vi "Set Test Window Topmost hacker.vi"(4 "error in (no error)":errorcluster, 7 "VI Refnum":refnum<vi>) -> (0 "error out":errorcluster, 1 "hWnd reference":T1, 2 "Window name":string, 3 "dup VI Refnum":refnum<vi>)   [LabVIEW 2011]
uses:
  SI.LIB/WIN32/WinUSER/Windows/hWnd.ctl
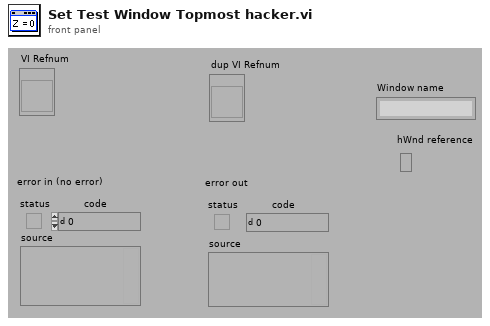
[diagram p1: front panel]
types:
  T1 = typedef "hWnd.ctl" = refnum<k1>
  T2 = enum32{"SW_SHOWDEFAULT", "SW_FORCEMINIMIZE", "SW_HIDE", "SW_MAXIMIZE", "SW_RESTORE", "SW_SHOW", "SW_SHOWMAXIMIZED", "SW_SHOWMINIMIZED", "SW_SHOWMINNOACTIVE", "SW_SHOWNA", "SW_SHOWNOACTIVATE", "SW_SHOWNORMAL"}
  T3 = cluster{"SWP_NOSIZE (x1)":bool, "SWP_NOMOVE (x2)":bool, "SWP_NOZORDER (x4)":bool, "SWP_NOREDRAW (x8)":bool, "SWP_NOACTIVATE (x10)":bool, "SWP_DRAWFRAME (x20)":bool, "SWP_SHOWWINDOW (x40)":bool, "SWP_HIDEWINDOW (x80)":bool, "SWP_NOCOPYBITS (x100)":bool, "SWP_NOOWNERZORDER (x200)":bool, "SWP_NOSENDCHANGING (x400)":bool, "SWP_DEFERERASE (x2000)":bool, "SWP_ASYNCWINDOWPOS (x4000)":bool}
  T4 = enum16{"HWND_TOP", "HWND_BOTTOM", "HWND_TOPMOST", "HWND_NOTOPMOST"}
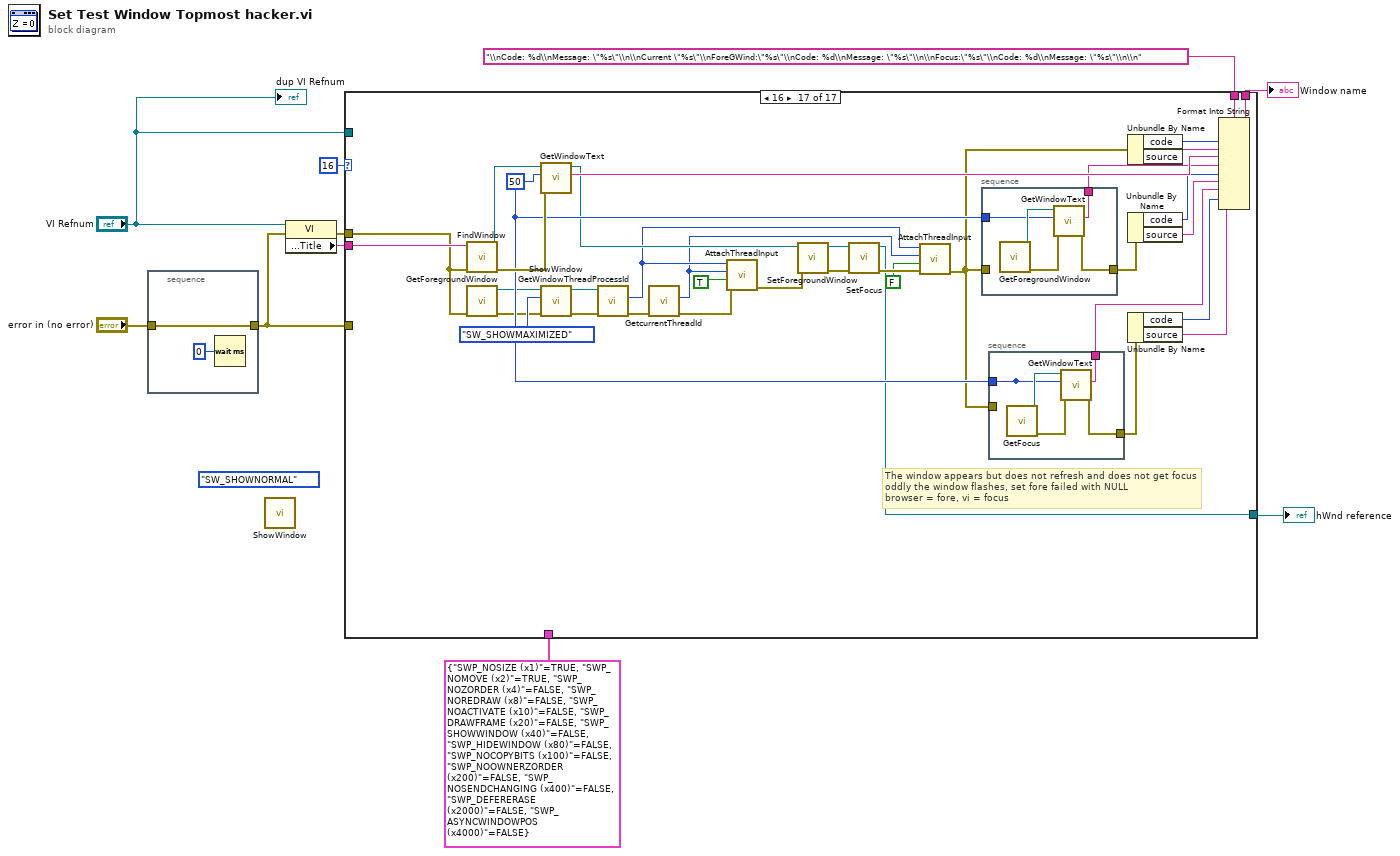
[diagram p0: block diagram]
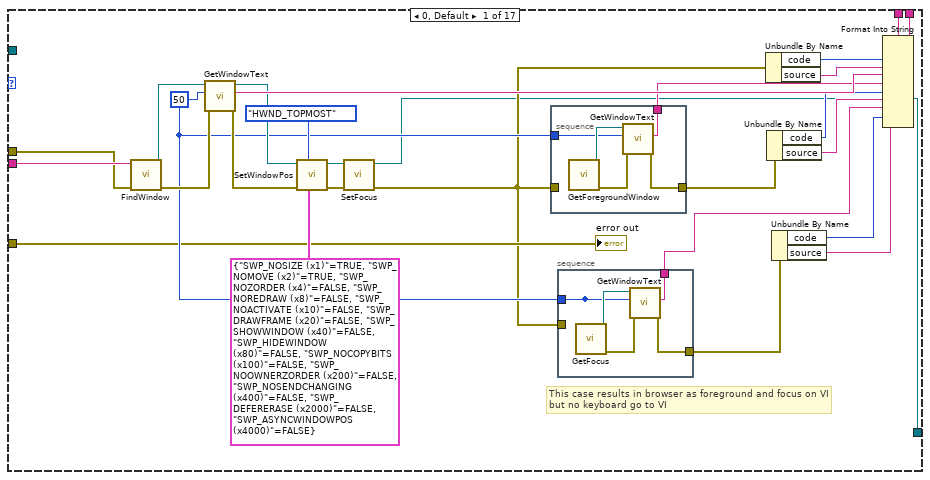
[diagram p2: hidden frame]
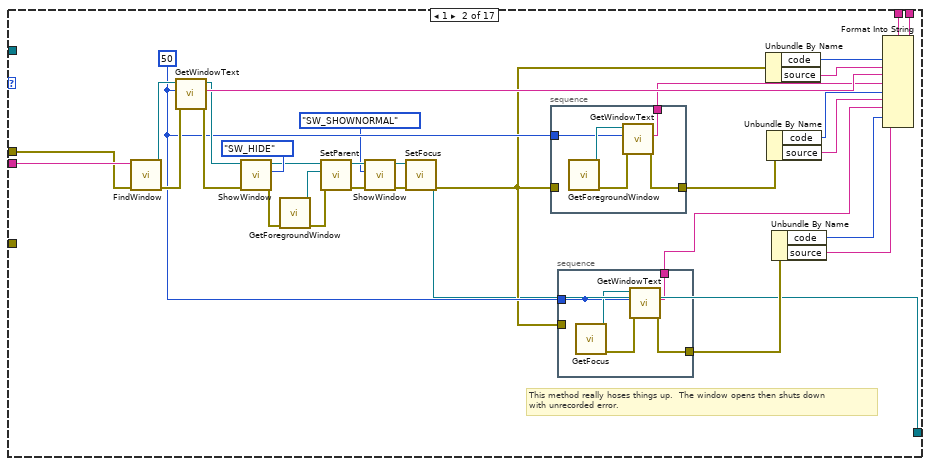
[diagram p3: hidden frame]
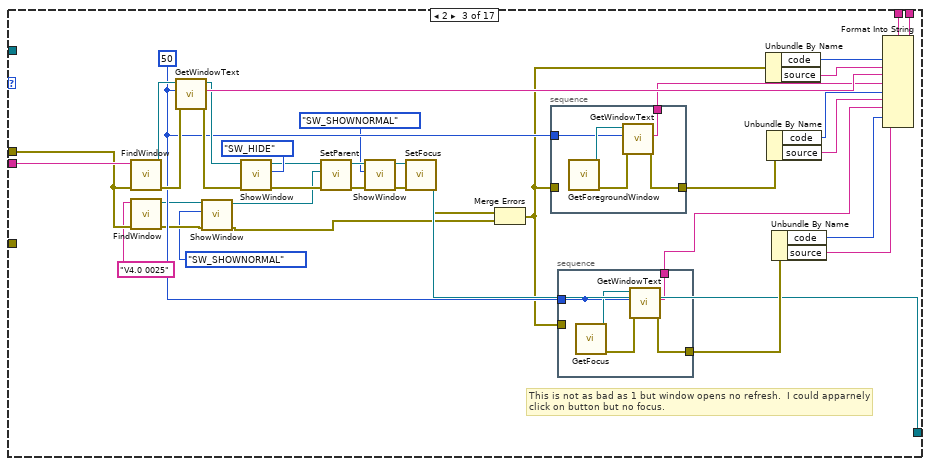
[diagram p4: hidden frame]
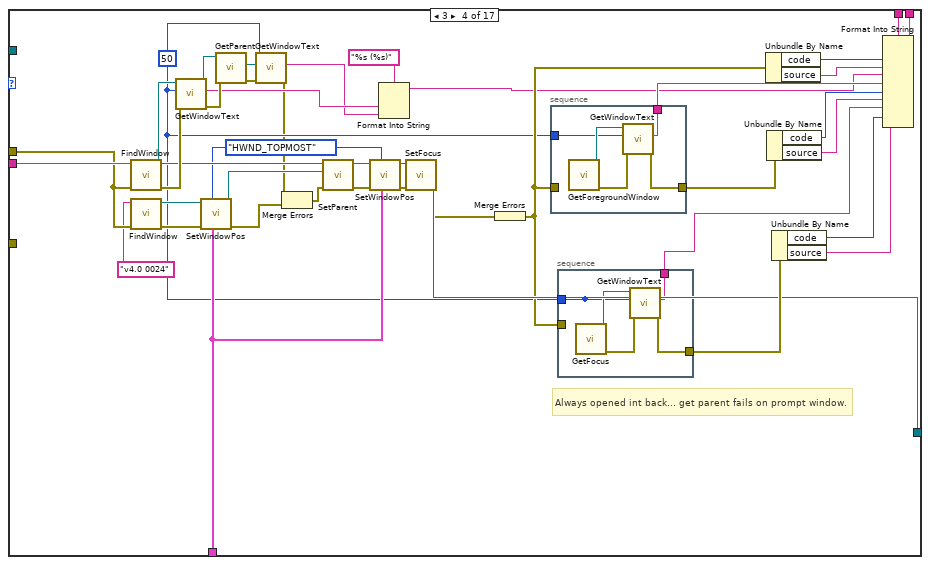
[diagram p5: hidden frame]
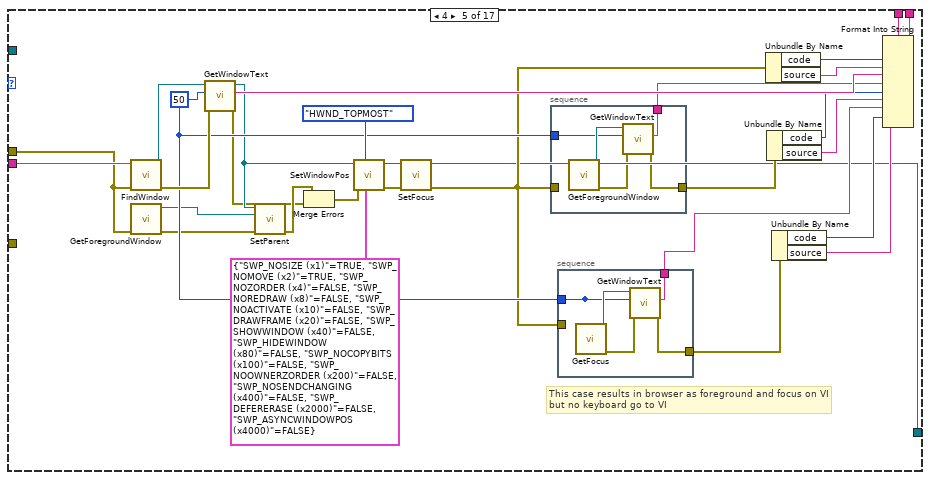
[diagram p6: hidden frame]
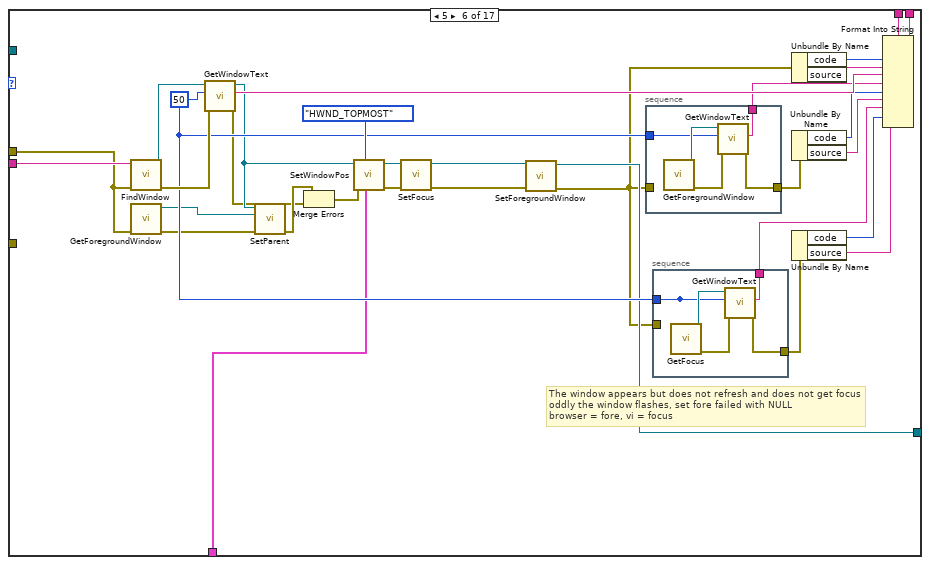
[diagram p7: hidden frame]
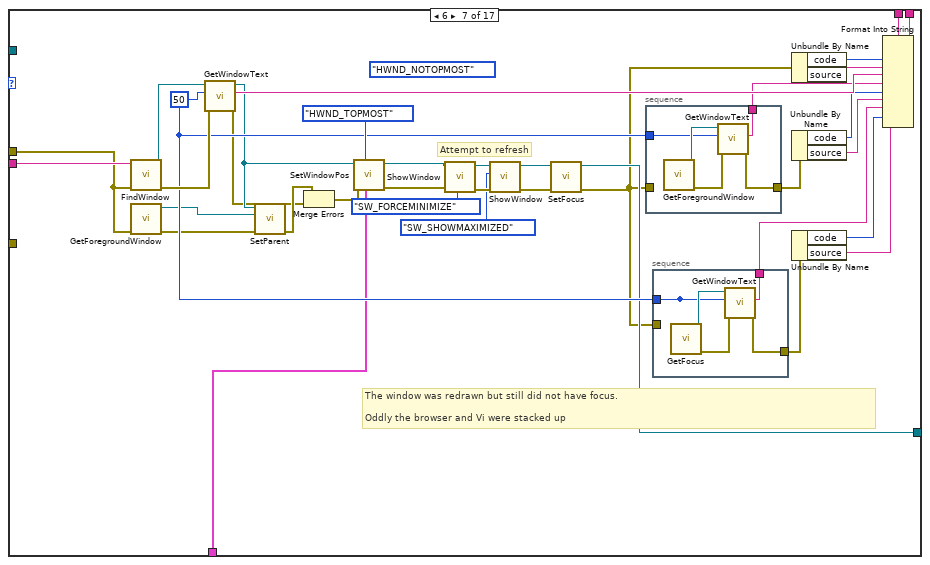
[diagram p8: hidden frame]
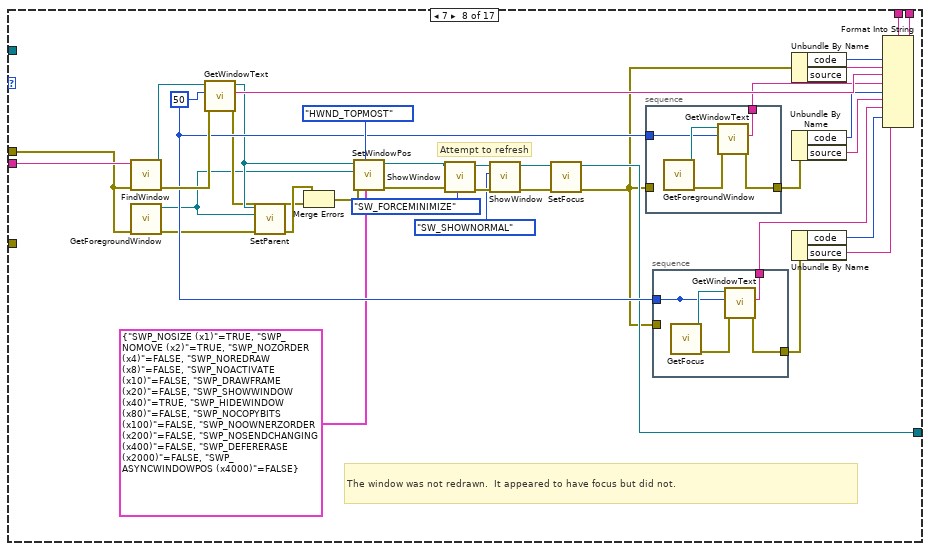
[diagram p9: hidden frame]
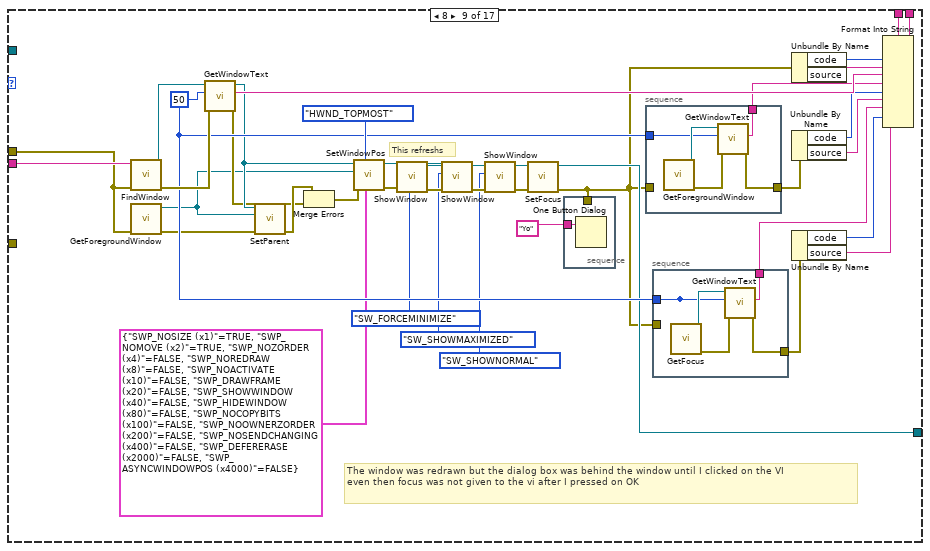
[diagram p10: hidden frame]
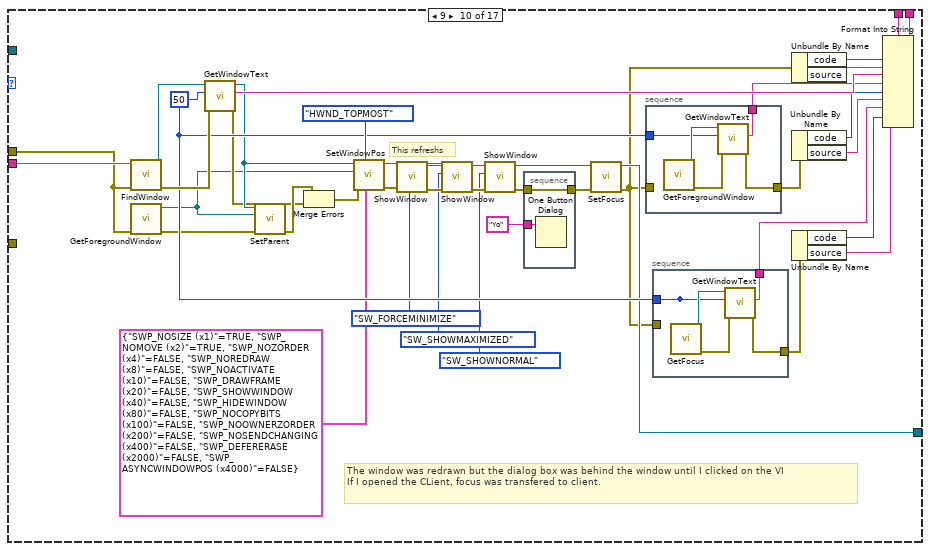
[diagram p11: hidden frame]
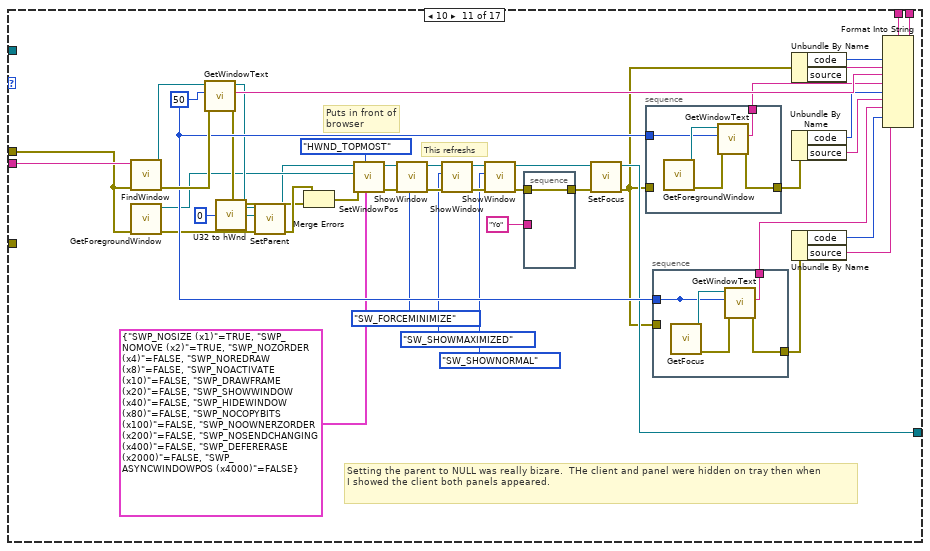
[diagram p12: hidden frame]
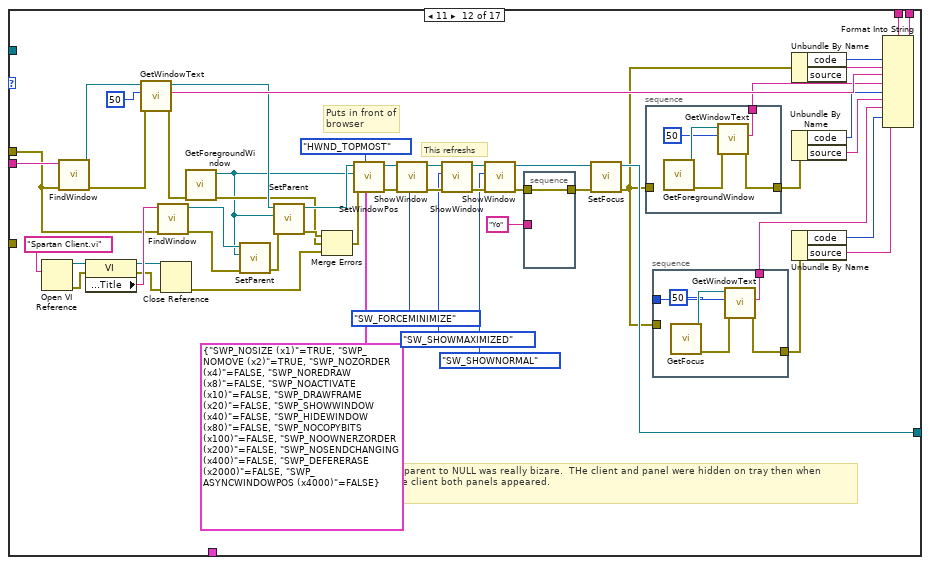
[diagram p13: hidden frame]
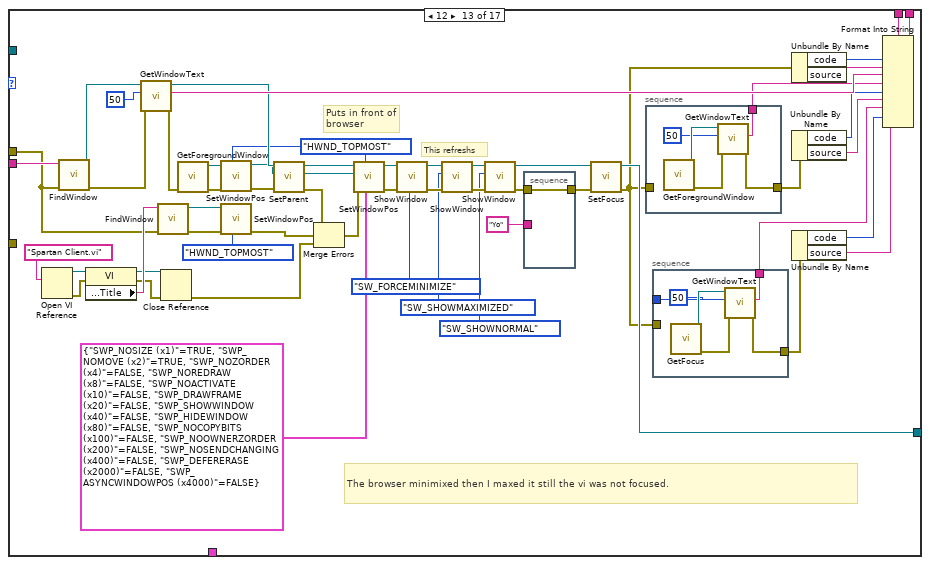
[diagram p14: hidden frame]
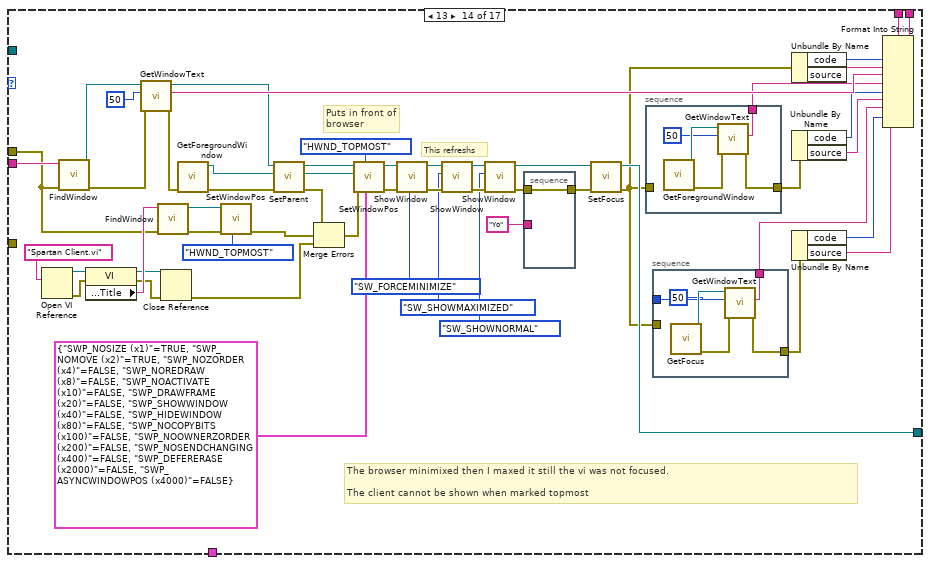
[diagram p15: hidden frame]
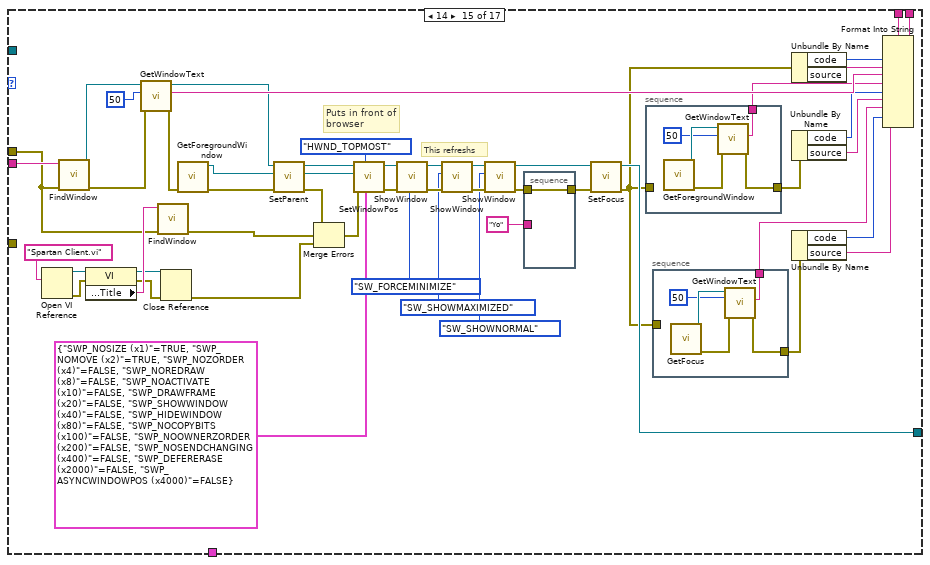
[diagram p16: hidden frame]
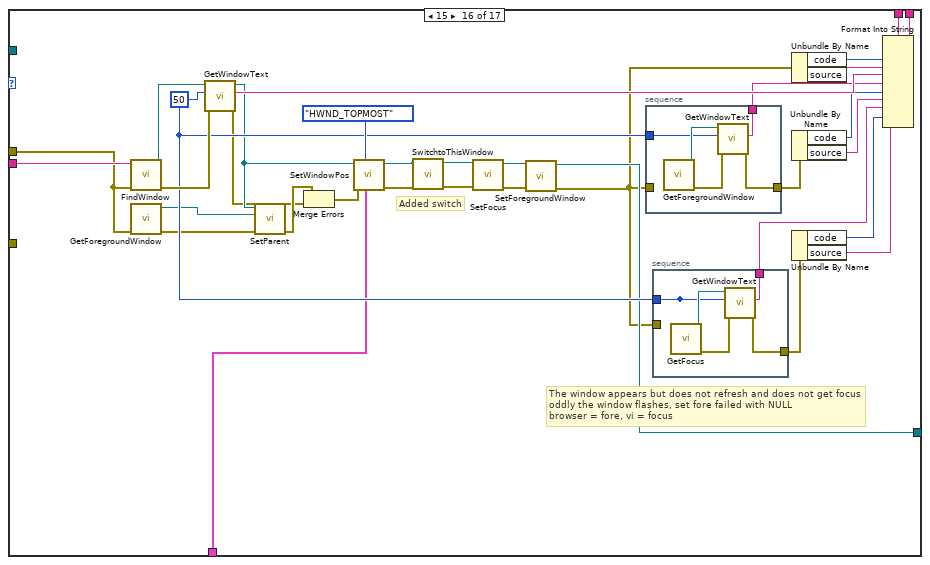
[diagram p17: hidden frame]
diagram:
  (unwired) T2."SW_SHOWNORMAL" ("nCmdShow\n(SW_SHOWNORMAL)")
  n1 = stacked-sequence {
    tunnel: "error in (no error)" -> [w12]
    tunnel: [w12] -> w5
    frame #0 {
      n2 = Wait (ms)(milliseconds to wait=u32 0) -> ()  [unwired: 1 out]
    }
  }
  n3 = call "ShowWindow.vi"() -> ()  [unwired: 4 in, 8 out]
  n4 = property class="VI"(reference="VI Refnum", error in=w5) -> (error out=w7:errorcluster, "Front Panel Window:Title"=w10:string)  [unwired: 1 out]
  n5 = case shown="16" 16 ("nMaxCount") {
    tunnel: w10 -> [w38 w81 w128 w179 w218 w261 w307 w353 w403 w455 w511 w574 w640 w704 w765 w810 w856]
    tunnel: "\\nCode: %d\\nMessage: \"%s\"\\n\\nCurrent \"%s\"\\nForeGWind:\"%s\"\\nCode: %d\\nMessage: \"%s\"\\n\\nFocus:\"%s\"\\nCode: %d\\nMessage: \"%s\"\\n\\n" ("format string") -> [w37 w80 w127 w178 w217 w260 w306 w352 w402 w454 w510 w573 w639 w703 w764 w809 w855]
    tunnel: [w36 w79 w126 w177 w216 w259 w305 w351 w401 w453 w509 w572 w638 w702 w763 w808 w854] -> w8
    tunnel: w7 -> [w34 w78 w101 w164 w196 w241 w289 w335 w385 w437 w493 w533 w601 w665 w726 w792 w839]
    tunnel: w5 -> [w15 _ _ _ _ _ _ _ _ _ _ _ _ _ _ _ _]
    tunnel: [w13 w60 w109 w165 w197 w231 w274 w322 w373 w425 w481 w547 w615 w679 w740 w782 w821] -> w4
    tunnel: T3 {"SWP_NOSIZE (x1)"=TRUE, "SWP_NOMOVE (x2)"=TRUE, "SWP_NOZORDER (x4)"=FALSE, "SWP_NOREDRAW (x8)"=FALSE, "SWP_NOACTIVATE (x10)"=FALSE, "SWP_DRAWFRAME (x20)"=FALSE, "SWP_SHOWWINDOW (x40)"=FALSE, "SWP_HIDEWINDOW (x80)"=FALSE, "SWP_NOCOPYBITS (x100)"=FALSE, "SWP_NOOWNERZORDER (x200)"=FALSE, "SWP_NOSENDCHANGING (x400)"=FALSE, "SWP_DEFERERASE (x2000)"=FALSE, "SWP_ASYNCWINDOWPOS (x4000)"=FALSE} ("Flags") -> [_ _ _ w151 _ w234 w282 _ _ _ _ _ _ _ _ w785 _]
    tunnel: "VI Refnum" -> [_ _ _ _ _ _ _ _ _ _ _ _ _ _ _ _ _]
    frame 0, Default {
      w21 = 50 ("nMaxCount")
      # "This case results in browser as foreground and focus on VI\nbut no keyboard go to VI"
      n6 = call "FindWindow.vi"("error in (no error)"=w34, "window name (\"\")"=w38) -> ("error out"=w30:errorcluster, "hWnd"=w25:T1)  [unwired: 6 out]
      n7 = call "GetWindowText.vi"("error in (no error)"=w30, "nMaxCount"=w21, "hWnd (NULL)"=w25) -> ("error out"=w29:errorcluster, "window text"=w31:string, "dup hWnd"=w27:T1)  [unwired: 6 out]
      n8 = call "SetWindowPos.vi"("Flags"=T3 {"SWP_NOSIZE (x1)"=TRUE, "SWP_NOMOVE (x2)"=TRUE, "SWP_NOZORDER (x4)"=FALSE, "SWP_NOREDRAW (x8)"=FALSE, "SWP_NOACTIVATE (x10)"=FALSE, "SWP_DRAWFRAME (x20)"=FALSE, "SWP_SHOWWINDOW (x40)"=FALSE, "SWP_HIDEWINDOW (x80)"=FALSE, "SWP_NOCOPYBITS (x100)"=FALSE, "SWP_NOOWNERZORDER (x200)"=FALSE, "SWP_NOSENDCHANGING (x400)"=FALSE, "SWP_DEFERERASE (x2000)"=FALSE, "SWP_ASYNCWINDOWPOS (x4000)"=FALSE}, "hWndInsertAfterALT\n(HWND_TOP)"=T4."HWND_TOPMOST" ("hWndInsertAfterALT\n(HWND_TOP)"), "error in (no error)"=w29, "hWnd (NULL)"=w27) -> ("error out"=w28:errorcluster, "dup hWnd"=w26:T1)  [unwired: 2 in, 4 out]
      n9 = call "SetFocus.vi"("error in (no error)"=w28, "hWnd (NULL)"=w26) -> ("error out"=w14:errorcluster, "dup hWnd"=w13:T1)  [unwired: 8 out]
      n10 = stacked-sequence {
        tunnel: w21 -> [w48]
        tunnel: [w46] -> w22
        tunnel: [w45] -> w16
        tunnel: w14 -> [_]
        frame #0 {
          n11 = call "GetForegroundWindow.vi"() -> ("error out"=w47:errorcluster, "dup hWnd"=w49:T1)  [unwired: 1 in, 9 out]
          n12 = call "GetWindowText.vi"("error in (no error)"=w47, "nMaxCount"=w48, "hWnd (NULL)"=w49) -> ("error out"=w45:errorcluster, "window text"=w46:string)  [unwired: 7 out]
        }
      }
      n13 = stacked-sequence {
        tunnel: [w40] -> _
        tunnel: [w42] -> w17
        tunnel: [w41] -> w20
        tunnel: w21 -> [w40]
        tunnel: w14 -> [_]
        frame #0 {
          n14 = call "GetFocus.vi"() -> ("error out"=w43:errorcluster, "dup hWnd"=w44:T1)  [unwired: 1 in, 9 out]
          n15 = call "GetWindowText.vi"("error in (no error)"=w43, "nMaxCount"=w40, "hWnd (NULL)"=w44) -> ("error out"=w41:errorcluster, "window text"=w42:string)  [unwired: 7 out]
        }
      }
      n16 = Unbundle By Name(w14) -> ("code"=w33:i32, "source"=w32:string)
      n17 = Unbundle By Name(w16) -> ("code"=w24:i32, "source"=w23:string)
      n18 = Unbundle By Name(w20) -> ("code"=w18:i32, "source"=w19:string)
      n19 = Format Into String(format string=w37, w33, w32, w31, w22, w24, w23, w17, w18, w19) -> (resulting string=w36:string)  [unwired: 2 in, 1 out]
      "error out" <- w15
    }
    frame 1 {
      w67 = 50 ("nMaxCount")
      # "This method really hoses things up.  The window opens then shuts down\nwith unrecorded error."
      n20 = call "FindWindow.vi"("error in (no error)"=w78, "window name (\"\")"=w81) -> ("error out"=w74:errorcluster, "hWnd"=w71:T1)  [unwired: 6 out]
      n21 = call "GetWindowText.vi"("error in (no error)"=w74, "nMaxCount"=w67, "hWnd (NULL)"=w71) -> ("error out"=w73:errorcluster, "window text"=w75:string, "dup hWnd"=w72:T1)  [unwired: 6 out]
      n22 = call "ShowWindow.vi"("error in (no error)"=w73, "nCmdShow\n(SW_SHOWNORMAL)"=T2."SW_HIDE" ("nCmdShow\n(SW_SHOWNORMAL)"), "hWnd (NULL)"=w72) -> ("error out"=w58:errorcluster, "dup hWnd"=w57:T1)  [unwired: 1 in, 6 out]
      n23 = call "GetForegroundWindow.vi"("error in (no error)"=w58) -> ("error out"=w55:errorcluster, "dup hWnd"=w56:T1)  [unwired: 9 out]
      n24 = call "SetParent.vi"("error in (no error)"=w55, "hWndParent (NULL)"=w56, "hWndChild (NULL)"=w57) -> ("error out"=w54:errorcluster, "dup hWndChild"=w53:T1)  [unwired: 7 out]
      n25 = call "ShowWindow.vi"("error in (no error)"=w54, "nCmdShow\n(SW_SHOWNORMAL)"=T2."SW_SHOWNORMAL" ("nCmdShow\n(SW_SHOWNORMAL)"), "hWnd (NULL)"=w53) -> ("error out"=w51:errorcluster, "dup hWnd"=w52:T1)  [unwired: 1 in, 6 out]
      n26 = call "SetFocus.vi"("error in (no error)"=w51, "hWnd (NULL)"=w52) -> ("error out"=w61:errorcluster, "dup hWnd"=w60:T1)  [unwired: 8 out]
      n27 = stacked-sequence {
        tunnel: w67 -> [w90]
        tunnel: [w88] -> w68
        tunnel: [w87] -> w62
        tunnel: w61 -> [_]
        frame #0 {
          n28 = call "GetForegroundWindow.vi"() -> ("error out"=w89:errorcluster, "dup hWnd"=w91:T1)  [unwired: 1 in, 9 out]
          n29 = call "GetWindowText.vi"("error in (no error)"=w89, "nMaxCount"=w90, "hWnd (NULL)"=w91) -> ("error out"=w87:errorcluster, "window text"=w88:string)  [unwired: 7 out]
        }
      }
      n30 = stacked-sequence {
        tunnel: [w82] -> _
        tunnel: [w84] -> w63
        tunnel: [w83] -> w66
        tunnel: w67 -> [w82]
        tunnel: w61 -> [_]
        frame #0 {
          n31 = call "GetFocus.vi"() -> ("error out"=w85:errorcluster, "dup hWnd"=w86:T1)  [unwired: 1 in, 9 out]
          n32 = call "GetWindowText.vi"("error in (no error)"=w85, "nMaxCount"=w82, "hWnd (NULL)"=w86) -> ("error out"=w83:errorcluster, "window text"=w84:string)  [unwired: 7 out]
        }
      }
      n33 = Unbundle By Name(w61) -> ("code"=w77:i32, "source"=w76:string)
      n34 = Unbundle By Name(w62) -> ("code"=w70:i32, "source"=w69:string)
      n35 = Unbundle By Name(w66) -> ("code"=w64:i32, "source"=w65:string)
      n36 = Format Into String(format string=w80, w77, w76, w75, w68, w70, w69, w63, w64, w65) -> (resulting string=w79:string)  [unwired: 2 in, 1 out]
    }
    frame 2 {
      w115 = 50 ("nMaxCount")
      # "This is not as bad as 1 but window opens no refresh.  I could apparnely\nclick on button but no focus."
      n37 = call "FindWindow.vi"("error in (no error)"=w101, "window name (\"\")"=w128) -> ("error out"=w122:errorcluster, "hWnd"=w119:T1)  [unwired: 6 out]
      n38 = call "FindWindow.vi"("error in (no error)"=w101, "window name (\"\")"="V4.0 0025") -> ("error out"=w97:errorcluster, "hWnd"=w98:T1)  [unwired: 6 out]
      n39 = call "GetWindowText.vi"("error in (no error)"=w122, "nMaxCount"=w115, "hWnd (NULL)"=w119) -> ("error out"=w121:errorcluster, "window text"=w123:string, "dup hWnd"=w120:T1)  [unwired: 6 out]
      n40 = call "ShowWindow.vi"("error in (no error)"=w97, "nCmdShow\n(SW_SHOWNORMAL)"=T2."SW_SHOWNORMAL" ("nCmdShow\n(SW_SHOWNORMAL)"), "hWnd (NULL)"=w98) -> ("error out"=w93:errorcluster, "dup hWnd"=w95:T1)  [unwired: 1 in, 6 out]
      n41 = call "ShowWindow.vi"("error in (no error)"=w121, "nCmdShow\n(SW_SHOWNORMAL)"=T2."SW_HIDE" ("nCmdShow\n(SW_SHOWNORMAL)"), "hWnd (NULL)"=w120) -> ("error out"=w99:errorcluster, "dup hWnd"=w107:T1)  [unwired: 1 in, 6 out]
      n42 = call "SetParent.vi"("error in (no error)"=w99, "hWndParent (NULL)"=w95, "hWndChild (NULL)"=w107) -> ("error out"=w106:errorcluster, "dup hWndChild"=w105:T1)  [unwired: 7 out]
      n43 = call "ShowWindow.vi"("error in (no error)"=w106, "nCmdShow\n(SW_SHOWNORMAL)"=T2."SW_SHOWNORMAL" ("nCmdShow\n(SW_SHOWNORMAL)"), "hWnd (NULL)"=w105) -> ("error out"=w103:errorcluster, "dup hWnd"=w104:T1)  [unwired: 1 in, 6 out]
      n44 = call "SetFocus.vi"("error in (no error)"=w103, "hWnd (NULL)"=w104) -> ("error out"=w94:errorcluster, "dup hWnd"=w109:T1)  [unwired: 8 out]
      n45 = Merge Errors(w94, w93) -> (w92:errorcluster)
      n46 = stacked-sequence {
        tunnel: w115 -> [w137]
        tunnel: [w135] -> w116
        tunnel: [w134] -> w110
        tunnel: w92 -> [_]
        frame #0 {
          n47 = call "GetForegroundWindow.vi"() -> ("error out"=w136:errorcluster, "dup hWnd"=w138:T1)  [unwired: 1 in, 9 out]
          n48 = call "GetWindowText.vi"("error in (no error)"=w136, "nMaxCount"=w137, "hWnd (NULL)"=w138) -> ("error out"=w134:errorcluster, "window text"=w135:string)  [unwired: 7 out]
        }
      }
      n49 = stacked-sequence {
        tunnel: [w129] -> _
        tunnel: [w131] -> w111
        tunnel: [w130] -> w114
        tunnel: w115 -> [w129]
        tunnel: w92 -> [_]
        frame #0 {
          n50 = call "GetFocus.vi"() -> ("error out"=w132:errorcluster, "dup hWnd"=w133:T1)  [unwired: 1 in, 9 out]
          n51 = call "GetWindowText.vi"("error in (no error)"=w132, "nMaxCount"=w129, "hWnd (NULL)"=w133) -> ("error out"=w130:errorcluster, "window text"=w131:string)  [unwired: 7 out]
        }
      }
      n52 = Unbundle By Name(w92) -> ("code"=w125:i32, "source"=w124:string)
      n53 = Unbundle By Name(w110) -> ("code"=w118:i32, "source"=w117:string)
      n54 = Unbundle By Name(w114) -> ("code"=w112:i32, "source"=w113:string)
      n55 = Format Into String(format string=w127, w125, w124, w123, w116, w118, w117, w111, w112, w113) -> (resulting string=w126:string)  [unwired: 2 in, 1 out]
    }
    frame 3 {
      w152 = T4."HWND_TOPMOST" ("hWndInsertAfterALT\n(HWND_TOP)")
      w147 = 50 ("nMaxCount")
      # "Always opened int back... get parent fails on prompt window."
      n56 = call "FindWindow.vi"("error in (no error)"=w164, "window name (\"\")"=w179) -> ("error out"=w174:errorcluster, "hWnd"=w159:T1)  [unwired: 6 out]
      n57 = call "FindWindow.vi"("error in (no error)"=w164, "window name (\"\")"="v4.0 0024") -> ("error out"=w160:errorcluster, "hWnd"=w157:T1)  [unwired: 6 out]
      n58 = call "GetWindowText.vi"("error in (no error)"=w174, "nMaxCount"=w147, "hWnd (NULL)"=w159) -> ("error out"=w149:errorcluster, "window text"=w144:string, "dup hWnd"=w150:T1)  [unwired: 6 out]
      n59 = call "SetWindowPos.vi"("Flags"=w151, "hWndInsertAfterALT\n(HWND_TOP)"=w152, "error in (no error)"=w160, "hWnd (NULL)"=w157) -> ("error out"=w140:errorcluster, "dup hWnd"=w158:T1)  [unwired: 2 in, 4 out]
      n60 = call "GetParent.vi"("error in (no error)"=w149, "hWndChild (NULL)"=w150) -> ("error out"=w142:errorcluster, "hWndParent"=w148:T1)  [unwired: 8 out]
      n61 = call "GetWindowText.vi"("error in (no error)"=w142, "nMaxCount"=w147, "hWnd (NULL)"=w148) -> ("error out"=w141:errorcluster, "window text"=w143:string)  [unwired: 7 out]
      n62 = Merge Errors(w141, w140) -> (w139:errorcluster)
      n63 = call "SetParent.vi"("error in (no error)"=w139, "hWndParent (NULL)"=w158, "hWndChild (NULL)"=w159) -> ("error out"=w156:errorcluster, "dup hWndChild"=w155:T1)  [unwired: 7 out]
      n64 = call "SetWindowPos.vi"("Flags"=w151, "hWndInsertAfterALT\n(HWND_TOP)"=w152, "error in (no error)"=w156, "hWnd (NULL)"=w155) -> ("error out"=w153:errorcluster, "dup hWnd"=w154:T1)  [unwired: 2 in, 4 out]
      n65 = Format Into String(format string="%s (%s)", w144, w143) -> (resulting string=w146:string)  [unwired: 2 in, 1 out]
      n66 = call "SetFocus.vi"("error in (no error)"=w153, "hWnd (NULL)"=w154) -> ("error out"=w162:errorcluster, "dup hWnd"=w165:T1)  [unwired: 8 out]
      n67 = Merge Errors(w162) -> (w161:errorcluster)
      n68 = stacked-sequence {
        tunnel: w147 -> [w188]
        tunnel: [w186] -> w171
        tunnel: [w185] -> w166
        tunnel: w161 -> [_]
        frame #0 {
          n69 = call "GetForegroundWindow.vi"() -> ("error out"=w187:errorcluster, "dup hWnd"=w189:T1)  [unwired: 1 in, 9 out]
          n70 = call "GetWindowText.vi"("error in (no error)"=w187, "nMaxCount"=w188, "hWnd (NULL)"=w189) -> ("error out"=w185:errorcluster, "window text"=w186:string)  [unwired: 7 out]
        }
      }
      n71 = stacked-sequence {
        tunnel: [w180] -> _
        tunnel: [w182] -> w167
        tunnel: [w181] -> w170
        tunnel: w147 -> [w180]
        tunnel: w161 -> [_]
        frame #0 {
          n72 = call "GetFocus.vi"() -> ("error out"=w183:errorcluster, "dup hWnd"=w184:T1)  [unwired: 1 in, 9 out]
          n73 = call "GetWindowText.vi"("error in (no error)"=w183, "nMaxCount"=w180, "hWnd (NULL)"=w184) -> ("error out"=w181:errorcluster, "window text"=w182:string)  [unwired: 7 out]
        }
      }
      n74 = Unbundle By Name(w161) -> ("code"=w176:i32, "source"=w175:string)
      n75 = Unbundle By Name(w166) -> ("code"=w173:i32, "source"=w172:string)
      n76 = Unbundle By Name(w170) -> ("code"=w168:i32, "source"=w169:string)
      n77 = Format Into String(format string=w178, w176, w175, w146, w171, w173, w172, w167, w168, w169) -> (resulting string=w177:string)  [unwired: 2 in, 1 out]
    }
    frame 4 {
      w204 = 50 ("nMaxCount")
      # "This case results in browser as foreground and focus on VI\nbut no keyboard go to VI"
      n78 = call "FindWindow.vi"("error in (no error)"=w196, "window name (\"\")"=w218) -> ("error out"=w211:errorcluster, "hWnd"=w208:T1)  [unwired: 6 out]
      n79 = call "GetForegroundWindow.vi"("error in (no error)"=w196) -> ("error out"=w195:errorcluster, "dup hWnd"=w194:T1)  [unwired: 9 out]
      n80 = call "GetWindowText.vi"("error in (no error)"=w211, "nMaxCount"=w204, "hWnd (NULL)"=w208) -> ("error out"=w191:errorcluster, "window text"=w212:string, "dup hWnd"=w193:T1)  [unwired: 6 out]
      n81 = call "SetParent.vi"("error in (no error)"=w195, "hWndParent (NULL)"=w194, "hWndChild (NULL)"=w193) -> ("error out"=w192:errorcluster)  [unwired: 8 out]
      n82 = Merge Errors(w192, w191) -> (w190:errorcluster)
      n83 = call "SetWindowPos.vi"("Flags"=T3 {"SWP_NOSIZE (x1)"=TRUE, "SWP_NOMOVE (x2)"=TRUE, "SWP_NOZORDER (x4)"=FALSE, "SWP_NOREDRAW (x8)"=FALSE, "SWP_NOACTIVATE (x10)"=FALSE, "SWP_DRAWFRAME (x20)"=FALSE, "SWP_SHOWWINDOW (x40)"=FALSE, "SWP_HIDEWINDOW (x80)"=FALSE, "SWP_NOCOPYBITS (x100)"=FALSE, "SWP_NOOWNERZORDER (x200)"=FALSE, "SWP_NOSENDCHANGING (x400)"=FALSE, "SWP_DEFERERASE (x2000)"=FALSE, "SWP_ASYNCWINDOWPOS (x4000)"=FALSE}, "hWndInsertAfterALT\n(HWND_TOP)"=T4."HWND_TOPMOST" ("hWndInsertAfterALT\n(HWND_TOP)"), "error in (no error)"=w190, "hWnd (NULL)"=w193) -> ("error out"=w210:errorcluster, "dup hWnd"=w209:T1)  [unwired: 2 in, 4 out]
      n84 = call "SetFocus.vi"("error in (no error)"=w210, "hWnd (NULL)"=w209) -> ("error out"=w198:errorcluster, "dup hWnd"=w197:T1)  [unwired: 8 out]
      n85 = stacked-sequence {
        tunnel: w204 -> [w228]
        tunnel: [w226] -> w205
        tunnel: [w225] -> w199
        tunnel: w198 -> [_]
        frame #0 {
          n86 = call "GetForegroundWindow.vi"() -> ("error out"=w227:errorcluster, "dup hWnd"=w229:T1)  [unwired: 1 in, 9 out]
          n87 = call "GetWindowText.vi"("error in (no error)"=w227, "nMaxCount"=w228, "hWnd (NULL)"=w229) -> ("error out"=w225:errorcluster, "window text"=w226:string)  [unwired: 7 out]
        }
      }
      n88 = stacked-sequence {
        tunnel: [w220] -> _
        tunnel: [w222] -> w200
        tunnel: [w221] -> w203
        tunnel: w204 -> [w220]
        tunnel: w198 -> [_]
        frame #0 {
          n89 = call "GetFocus.vi"() -> ("error out"=w223:errorcluster, "dup hWnd"=w224:T1)  [unwired: 1 in, 9 out]
          n90 = call "GetWindowText.vi"("error in (no error)"=w223, "nMaxCount"=w220, "hWnd (NULL)"=w224) -> ("error out"=w221:errorcluster, "window text"=w222:string)  [unwired: 7 out]
        }
      }
      n91 = Unbundle By Name(w198) -> ("code"=w214:i32, "source"=w213:string)
      n92 = Unbundle By Name(w199) -> ("code"=w207:i32, "source"=w206:string)
      n93 = Unbundle By Name(w203) -> ("code"=w201:i32, "source"=w202:string)
      n94 = Format Into String(format string=w217, w214, w213, w212, w205, w207, w206, w200, w201, w202) -> (resulting string=w216:string)  [unwired: 2 in, 1 out]
    }
    frame 5 {
      w247 = 50 ("nMaxCount")
      # "The window appears but does not refresh and does not get focus\noddly the window flashes, set fore failed with NULL\nbrowser = fore, vi = focus"
      n95 = call "FindWindow.vi"("error in (no error)"=w241, "window name (\"\")"=w261) -> ("error out"=w254:errorcluster, "hWnd"=w251:T1)  [unwired: 6 out]
      n96 = call "GetForegroundWindow.vi"("error in (no error)"=w241) -> ("error out"=w240:errorcluster, "dup hWnd"=w239:T1)  [unwired: 9 out]
      n97 = call "GetWindowText.vi"("error in (no error)"=w254, "nMaxCount"=w247, "hWnd (NULL)"=w251) -> ("error out"=w236:errorcluster, "window text"=w255:string, "dup hWnd"=w238:T1)  [unwired: 6 out]
      n98 = call "SetParent.vi"("error in (no error)"=w240, "hWndParent (NULL)"=w239, "hWndChild (NULL)"=w238) -> ("error out"=w237:errorcluster)  [unwired: 8 out]
      n99 = Merge Errors(w237, w236) -> (w235:errorcluster)
      n100 = call "SetWindowPos.vi"("Flags"=w234, "hWndInsertAfterALT\n(HWND_TOP)"=T4."HWND_TOPMOST" ("hWndInsertAfterALT\n(HWND_TOP)"), "error in (no error)"=w235, "hWnd (NULL)"=w238) -> ("error out"=w253:errorcluster, "dup hWnd"=w252:T1)  [unwired: 2 in, 4 out]
      n101 = call "SetFocus.vi"("error in (no error)"=w253, "hWnd (NULL)"=w252) -> ("error out"=w233:errorcluster, "dup hWnd"=w232:T1)  [unwired: 8 out]
      n102 = call "SetForegroundWindow.vi"("error in (no error)"=w233, "hWnd (NULL)"=w232) -> ("error out"=w230:errorcluster, "dup hWnd"=w231:T1)  [unwired: 8 out]
      n103 = stacked-sequence {
        tunnel: w247 -> [w270]
        tunnel: [w268] -> w248
        tunnel: [w267] -> w242
        tunnel: w230 -> [_]
        frame #0 {
          n104 = call "GetForegroundWindow.vi"() -> ("error out"=w269:errorcluster, "dup hWnd"=w271:T1)  [unwired: 1 in, 9 out]
          n105 = call "GetWindowText.vi"("error in (no error)"=w269, "nMaxCount"=w270, "hWnd (NULL)"=w271) -> ("error out"=w267:errorcluster, "window text"=w268:string)  [unwired: 7 out]
        }
      }
      n106 = stacked-sequence {
        tunnel: [w262] -> _
        tunnel: [w264] -> w243
        tunnel: [w263] -> w246
        tunnel: w247 -> [w262]
        tunnel: w230 -> [_]
        frame #0 {
          n107 = call "GetFocus.vi"() -> ("error out"=w265:errorcluster, "dup hWnd"=w266:T1)  [unwired: 1 in, 9 out]
          n108 = call "GetWindowText.vi"("error in (no error)"=w265, "nMaxCount"=w262, "hWnd (NULL)"=w266) -> ("error out"=w263:errorcluster, "window text"=w264:string)  [unwired: 7 out]
        }
      }
      n109 = Unbundle By Name(w230) -> ("code"=w257:i32, "source"=w256:string)
      n110 = Unbundle By Name(w242) -> ("code"=w250:i32, "source"=w249:string)
      n111 = Unbundle By Name(w246) -> ("code"=w244:i32, "source"=w245:string)
      n112 = Format Into String(format string=w260, w257, w256, w255, w248, w250, w249, w243, w244, w245) -> (resulting string=w259:string)  [unwired: 2 in, 1 out]
    }
    frame 6 {
      (unwired) T4."HWND_NOTOPMOST" ("hWndInsertAfterALT\n(HWND_TOP)")
      w295 = 50 ("nMaxCount")
      # "The window was redrawn but still did not have focus.\n\nOddly the browser and Vi were stacked up"
      # "Attempt to refresh"
      n113 = call "FindWindow.vi"("error in (no error)"=w289, "window name (\"\")"=w307) -> ("error out"=w300:errorcluster, "hWnd"=w299:T1)  [unwired: 6 out]
      n114 = call "GetForegroundWindow.vi"("error in (no error)"=w289) -> ("error out"=w288:errorcluster, "dup hWnd"=w287:T1)  [unwired: 9 out]
      n115 = call "GetWindowText.vi"("error in (no error)"=w300, "nMaxCount"=w295, "hWnd (NULL)"=w299) -> ("error out"=w284:errorcluster, "window text"=w301:string, "dup hWnd"=w286:T1)  [unwired: 6 out]
      n116 = call "SetParent.vi"("error in (no error)"=w288, "hWndParent (NULL)"=w287, "hWndChild (NULL)"=w286) -> ("error out"=w285:errorcluster)  [unwired: 8 out]
      n117 = Merge Errors(w285, w284) -> (w283:errorcluster)
      n118 = call "SetWindowPos.vi"("Flags"=w282, "hWndInsertAfterALT\n(HWND_TOP)"=T4."HWND_TOPMOST" ("hWndInsertAfterALT\n(HWND_TOP)"), "error in (no error)"=w283, "hWnd (NULL)"=w286) -> ("error out"=w276:errorcluster, "dup hWnd"=w277:T1)  [unwired: 2 in, 4 out]
      n119 = call "ShowWindow.vi"("error in (no error)"=w276, "nCmdShow\n(SW_SHOWNORMAL)"=T2."SW_FORCEMINIMIZE" ("nCmdShow\n(SW_SHOWNORMAL)"), "hWnd (NULL)"=w277) -> ("error out"=w281:errorcluster, "dup hWnd"=w280:T1)  [unwired: 7 out]
      n120 = call "ShowWindow.vi"("error in (no error)"=w281, "nCmdShow\n(SW_SHOWNORMAL)"=T2."SW_SHOWMAXIMIZED" ("nCmdShow\n(SW_SHOWNORMAL)"), "hWnd (NULL)"=w280) -> ("error out"=w273:errorcluster, "dup hWnd"=w275:T1)  [unwired: 7 out]
      n121 = call "SetFocus.vi"("error in (no error)"=w273, "hWnd (NULL)"=w275) -> ("error out"=w272:errorcluster, "dup hWnd"=w274:T1)  [unwired: 8 out]
      n122 = stacked-sequence {
        tunnel: w295 -> [w316]
        tunnel: [w314] -> w296
        tunnel: [w313] -> w290
        tunnel: w272 -> [_]
        frame #0 {
          n123 = call "GetForegroundWindow.vi"() -> ("error out"=w315:errorcluster, "dup hWnd"=w317:T1)  [unwired: 1 in, 9 out]
          n124 = call "GetWindowText.vi"("error in (no error)"=w315, "nMaxCount"=w316, "hWnd (NULL)"=w317) -> ("error out"=w313:errorcluster, "window text"=w314:string)  [unwired: 7 out]
        }
      }
      n125 = stacked-sequence {
        tunnel: [w308] -> _
        tunnel: [w310] -> w291
        tunnel: [w309] -> w294
        tunnel: w295 -> [w308]
        tunnel: w272 -> [_]
        frame #0 {
          n126 = call "GetFocus.vi"() -> ("error out"=w311:errorcluster, "dup hWnd"=w312:T1)  [unwired: 1 in, 9 out]
          n127 = call "GetWindowText.vi"("error in (no error)"=w311, "nMaxCount"=w308, "hWnd (NULL)"=w312) -> ("error out"=w309:errorcluster, "window text"=w310:string)  [unwired: 7 out]
        }
      }
      n128 = Unbundle By Name(w272) -> ("code"=w303:i32, "source"=w302:string)
      n129 = Unbundle By Name(w290) -> ("code"=w298:i32, "source"=w297:string)
      n130 = Unbundle By Name(w294) -> ("code"=w292:i32, "source"=w293:string)
      n131 = Format Into String(format string=w306, w303, w302, w301, w296, w298, w297, w291, w292, w293) -> (resulting string=w305:string)  [unwired: 2 in, 1 out]
    }
    frame 7 {
      w341 = 50 ("nMaxCount")
      # "The window was not redrawn.  It appeared to have focus but did not."
      # "Attempt to refresh"
      n132 = call "FindWindow.vi"("error in (no error)"=w335, "window name (\"\")"=w353) -> ("error out"=w346:errorcluster, "hWnd"=w345:T1)  [unwired: 6 out]
      n133 = call "GetForegroundWindow.vi"("error in (no error)"=w335) -> ("error out"=w334:errorcluster, "dup hWnd"=w318:T1)  [unwired: 9 out]
      n134 = call "GetWindowText.vi"("error in (no error)"=w346, "nMaxCount"=w341, "hWnd (NULL)"=w345) -> ("error out"=w331:errorcluster, "window text"=w347:string, "dup hWnd"=w333:T1)  [unwired: 6 out]
      n135 = call "SetParent.vi"("error in (no error)"=w334, "hWndParent (NULL)"=w318, "hWndChild (NULL)"=w333) -> ("error out"=w332:errorcluster)  [unwired: 8 out]
      n136 = Merge Errors(w332, w331) -> (w330:errorcluster)
      n137 = call "SetWindowPos.vi"("Flags"=T3 {"SWP_NOSIZE (x1)"=TRUE, "SWP_NOMOVE (x2)"=TRUE, "SWP_NOZORDER (x4)"=FALSE, "SWP_NOREDRAW (x8)"=FALSE, "SWP_NOACTIVATE (x10)"=FALSE, "SWP_DRAWFRAME (x20)"=FALSE, "SWP_SHOWWINDOW (x40)"=TRUE, "SWP_HIDEWINDOW (x80)"=FALSE, "SWP_NOCOPYBITS (x100)"=FALSE, "SWP_NOOWNERZORDER (x200)"=FALSE, "SWP_NOSENDCHANGING (x400)"=FALSE, "SWP_DEFERERASE (x2000)"=FALSE, "SWP_ASYNCWINDOWPOS (x4000)"=FALSE}, "hWndInsertAfterALT\n(HWND_TOP)"=T4."HWND_TOPMOST" ("hWndInsertAfterALT\n(HWND_TOP)"), "error in (no error)"=w330, "hWndInsertAfter\n(NULL - use ALT)"=w318, "hWnd (NULL)"=w333) -> ("error out"=w324:errorcluster, "dup hWnd"=w325:T1)  [unwired: 1 in, 4 out]
      n138 = call "ShowWindow.vi"("error in (no error)"=w324, "nCmdShow\n(SW_SHOWNORMAL)"=T2."SW_FORCEMINIMIZE" ("nCmdShow\n(SW_SHOWNORMAL)"), "hWnd (NULL)"=w325) -> ("error out"=w329:errorcluster, "dup hWnd"=w328:T1)  [unwired: 7 out]
      n139 = call "ShowWindow.vi"("error in (no error)"=w329, "nCmdShow\n(SW_SHOWNORMAL)"=T2."SW_SHOWNORMAL" ("nCmdShow\n(SW_SHOWNORMAL)"), "hWnd (NULL)"=w328) -> ("error out"=w321:errorcluster, "dup hWnd"=w323:T1)  [unwired: 7 out]
      n140 = call "SetFocus.vi"("error in (no error)"=w321, "hWnd (NULL)"=w323) -> ("error out"=w320:errorcluster, "dup hWnd"=w322:T1)  [unwired: 8 out]
      n141 = stacked-sequence {
        tunnel: w341 -> [w362]
        tunnel: [w360] -> w342
        tunnel: [w359] -> w336
        tunnel: w320 -> [_]
        frame #0 {
          n142 = call "GetForegroundWindow.vi"() -> ("error out"=w361:errorcluster, "dup hWnd"=w363:T1)  [unwired: 1 in, 9 out]
          n143 = call "GetWindowText.vi"("error in (no error)"=w361, "nMaxCount"=w362, "hWnd (NULL)"=w363) -> ("error out"=w359:errorcluster, "window text"=w360:string)  [unwired: 7 out]
        }
      }
      n144 = stacked-sequence {
        tunnel: [w354] -> _
        tunnel: [w356] -> w337
        tunnel: [w355] -> w340
        tunnel: w341 -> [w354]
        tunnel: w320 -> [_]
        frame #0 {
          n145 = call "GetFocus.vi"() -> ("error out"=w357:errorcluster, "dup hWnd"=w358:T1)  [unwired: 1 in, 9 out]
          n146 = call "GetWindowText.vi"("error in (no error)"=w357, "nMaxCount"=w354, "hWnd (NULL)"=w358) -> ("error out"=w355:errorcluster, "window text"=w356:string)  [unwired: 7 out]
        }
      }
      n147 = Unbundle By Name(w320) -> ("code"=w349:i32, "source"=w348:string)
      n148 = Unbundle By Name(w336) -> ("code"=w344:i32, "source"=w343:string)
      n149 = Unbundle By Name(w340) -> ("code"=w338:i32, "source"=w339:string)
      n150 = Format Into String(format string=w352, w349, w348, w347, w342, w344, w343, w337, w338, w339) -> (resulting string=w351:string)  [unwired: 2 in, 1 out]
    }
    frame 8 {
      w391 = 50 ("nMaxCount")
      # "The window was redrawn but the dialog box was behind the window until I clicked on the VI\neven then focus was not given to the vi after I pressed on OK"
      # "This refreshs"
      n151 = call "FindWindow.vi"("error in (no error)"=w385, "window name (\"\")"=w403) -> ("error out"=w396:errorcluster, "hWnd"=w395:T1)  [unwired: 6 out]
      n152 = call "GetForegroundWindow.vi"("error in (no error)"=w385) -> ("error out"=w384:errorcluster, "dup hWnd"=w371:T1)  [unwired: 9 out]
      n153 = call "GetWindowText.vi"("error in (no error)"=w396, "nMaxCount"=w391, "hWnd (NULL)"=w395) -> ("error out"=w381:errorcluster, "window text"=w397:string, "dup hWnd"=w383:T1)  [unwired: 6 out]
      n154 = call "SetParent.vi"("error in (no error)"=w384, "hWndParent (NULL)"=w371, "hWndChild (NULL)"=w383) -> ("error out"=w382:errorcluster)  [unwired: 8 out]
      n155 = Merge Errors(w382, w381) -> (w380:errorcluster)
      n156 = call "SetWindowPos.vi"("Flags"=T3 {"SWP_NOSIZE (x1)"=TRUE, "SWP_NOMOVE (x2)"=TRUE, "SWP_NOZORDER (x4)"=FALSE, "SWP_NOREDRAW (x8)"=FALSE, "SWP_NOACTIVATE (x10)"=FALSE, "SWP_DRAWFRAME (x20)"=FALSE, "SWP_SHOWWINDOW (x40)"=FALSE, "SWP_HIDEWINDOW (x80)"=FALSE, "SWP_NOCOPYBITS (x100)"=FALSE, "SWP_NOOWNERZORDER (x200)"=FALSE, "SWP_NOSENDCHANGING (x400)"=FALSE, "SWP_DEFERERASE (x2000)"=FALSE, "SWP_ASYNCWINDOWPOS (x4000)"=FALSE}, "hWndInsertAfterALT\n(HWND_TOP)"=T4."HWND_TOPMOST" ("hWndInsertAfterALT\n(HWND_TOP)"), "error in (no error)"=w380, "hWndInsertAfter\n(NULL - use ALT)"=w371, "hWnd (NULL)"=w383) -> ("error out"=w374:errorcluster, "dup hWnd"=w375:T1)  [unwired: 1 in, 4 out]
      n157 = call "ShowWindow.vi"("error in (no error)"=w374, "nCmdShow\n(SW_SHOWNORMAL)"=T2."SW_FORCEMINIMIZE" ("nCmdShow\n(SW_SHOWNORMAL)"), "hWnd (NULL)"=w375) -> ("error out"=w379:errorcluster, "dup hWnd"=w378:T1)  [unwired: 7 out]
      n158 = call "ShowWindow.vi"("error in (no error)"=w379, "nCmdShow\n(SW_SHOWNORMAL)"=T2."SW_SHOWMAXIMIZED" ("nCmdShow\n(SW_SHOWNORMAL)"), "hWnd (NULL)"=w378) -> ("error out"=w368:errorcluster, "dup hWnd"=w370:T1)  [unwired: 7 out]
      n159 = call "ShowWindow.vi"("error in (no error)"=w368, "nCmdShow\n(SW_SHOWNORMAL)"=T2."SW_SHOWNORMAL" ("nCmdShow\n(SW_SHOWNORMAL)"), "hWnd (NULL)"=w370) -> ("error out"=w367:errorcluster, "dup hWnd"=w369:T1)  [unwired: 7 out]
      n160 = call "SetFocus.vi"("error in (no error)"=w367, "hWnd (NULL)"=w369) -> ("error out"=w365:errorcluster, "dup hWnd"=w373:T1)  [unwired: 8 out]
      n161 = stacked-sequence {
        tunnel: w365 -> [_]
        tunnel: "Yo" -> [w404]
        frame #0 {
          n162 = One Button Dialog(message=w404) -> ()  [unwired: 2 out]
        }
      }
      n163 = stacked-sequence {
        tunnel: w391 -> [w413]
        tunnel: [w411] -> w392
        tunnel: [w410] -> w386
        tunnel: w365 -> [_]
        frame #0 {
          n164 = call "GetForegroundWindow.vi"() -> ("error out"=w412:errorcluster, "dup hWnd"=w414:T1)  [unwired: 1 in, 9 out]
          n165 = call "GetWindowText.vi"("error in (no error)"=w412, "nMaxCount"=w413, "hWnd (NULL)"=w414) -> ("error out"=w410:errorcluster, "window text"=w411:string)  [unwired: 7 out]
        }
      }
      n166 = stacked-sequence {
        tunnel: [w405] -> _
        tunnel: [w407] -> w387
        tunnel: [w406] -> w390
        tunnel: w391 -> [w405]
        tunnel: w365 -> [_]
        frame #0 {
          n167 = call "GetFocus.vi"() -> ("error out"=w408:errorcluster, "dup hWnd"=w409:T1)  [unwired: 1 in, 9 out]
          n168 = call "GetWindowText.vi"("error in (no error)"=w408, "nMaxCount"=w405, "hWnd (NULL)"=w409) -> ("error out"=w406:errorcluster, "window text"=w407:string)  [unwired: 7 out]
        }
      }
      n169 = Unbundle By Name(w365) -> ("code"=w399:i32, "source"=w398:string)
      n170 = Unbundle By Name(w386) -> ("code"=w394:i32, "source"=w393:string)
      n171 = Unbundle By Name(w390) -> ("code"=w388:i32, "source"=w389:string)
      n172 = Format Into String(format string=w402, w399, w398, w397, w392, w394, w393, w387, w388, w389) -> (resulting string=w401:string)  [unwired: 2 in, 1 out]
    }
    frame 9 {
      w443 = 50 ("nMaxCount")
      # "The window was redrawn but the dialog box was behind the window until I clicked on the VI\nIf I opened the CLient, focus was transfered to client."
      # "This refreshs"
      n173 = call "FindWindow.vi"("error in (no error)"=w437, "window name (\"\")"=w455) -> ("error out"=w448:errorcluster, "hWnd"=w447:T1)  [unwired: 6 out]
      n174 = call "GetForegroundWindow.vi"("error in (no error)"=w437) -> ("error out"=w436:errorcluster, "dup hWnd"=w423:T1)  [unwired: 9 out]
      n175 = call "GetWindowText.vi"("error in (no error)"=w448, "nMaxCount"=w443, "hWnd (NULL)"=w447) -> ("error out"=w433:errorcluster, "window text"=w449:string, "dup hWnd"=w435:T1)  [unwired: 6 out]
      n176 = call "SetParent.vi"("error in (no error)"=w436, "hWndParent (NULL)"=w423, "hWndChild (NULL)"=w435) -> ("error out"=w434:errorcluster)  [unwired: 8 out]
      n177 = Merge Errors(w434, w433) -> (w432:errorcluster)
      n178 = call "SetWindowPos.vi"("Flags"=T3 {"SWP_NOSIZE (x1)"=TRUE, "SWP_NOMOVE (x2)"=TRUE, "SWP_NOZORDER (x4)"=FALSE, "SWP_NOREDRAW (x8)"=FALSE, "SWP_NOACTIVATE (x10)"=FALSE, "SWP_DRAWFRAME (x20)"=FALSE, "SWP_SHOWWINDOW (x40)"=FALSE, "SWP_HIDEWINDOW (x80)"=FALSE, "SWP_NOCOPYBITS (x100)"=FALSE, "SWP_NOOWNERZORDER (x200)"=FALSE, "SWP_NOSENDCHANGING (x400)"=FALSE, "SWP_DEFERERASE (x2000)"=FALSE, "SWP_ASYNCWINDOWPOS (x4000)"=FALSE}, "hWndInsertAfterALT\n(HWND_TOP)"=T4."HWND_TOPMOST" ("hWndInsertAfterALT\n(HWND_TOP)"), "error in (no error)"=w432, "hWndInsertAfter\n(NULL - use ALT)"=w423, "hWnd (NULL)"=w435) -> ("error out"=w426:errorcluster, "dup hWnd"=w427:T1)  [unwired: 1 in, 4 out]
      n179 = call "ShowWindow.vi"("error in (no error)"=w426, "nCmdShow\n(SW_SHOWNORMAL)"=T2."SW_FORCEMINIMIZE" ("nCmdShow\n(SW_SHOWNORMAL)"), "hWnd (NULL)"=w427) -> ("error out"=w431:errorcluster, "dup hWnd"=w430:T1)  [unwired: 7 out]
      n180 = call "ShowWindow.vi"("error in (no error)"=w431, "nCmdShow\n(SW_SHOWNORMAL)"=T2."SW_SHOWMAXIMIZED" ("nCmdShow\n(SW_SHOWNORMAL)"), "hWnd (NULL)"=w430) -> ("error out"=w420:errorcluster, "dup hWnd"=w422:T1)  [unwired: 7 out]
      n181 = call "ShowWindow.vi"("error in (no error)"=w420, "nCmdShow\n(SW_SHOWNORMAL)"=T2."SW_SHOWNORMAL" ("nCmdShow\n(SW_SHOWNORMAL)"), "hWnd (NULL)"=w422) -> ("error out"=w416:errorcluster, "dup hWnd"=w421:T1)  [unwired: 7 out]
      n182 = stacked-sequence {
        tunnel: "Yo" -> [w457]
        tunnel: w416 -> [w456]
        tunnel: [w456] -> w415
        frame #0 {
          n183 = One Button Dialog(message=w457) -> ()  [unwired: 2 out]
        }
      }
      n184 = call "SetFocus.vi"("error in (no error)"=w415, "hWnd (NULL)"=w421) -> ("error out"=w418:errorcluster, "dup hWnd"=w425:T1)  [unwired: 8 out]
      n185 = stacked-sequence {
        tunnel: w443 -> [w466]
        tunnel: [w464] -> w444
        tunnel: [w463] -> w438
        tunnel: w418 -> [_]
        frame #0 {
          n186 = call "GetForegroundWindow.vi"() -> ("error out"=w465:errorcluster, "dup hWnd"=w467:T1)  [unwired: 1 in, 9 out]
          n187 = call "GetWindowText.vi"("error in (no error)"=w465, "nMaxCount"=w466, "hWnd (NULL)"=w467) -> ("error out"=w463:errorcluster, "window text"=w464:string)  [unwired: 7 out]
        }
      }
      n188 = stacked-sequence {
        tunnel: [w458] -> _
        tunnel: [w460] -> w439
        tunnel: [w459] -> w442
        tunnel: w443 -> [w458]
        tunnel: w418 -> [_]
        frame #0 {
          n189 = call "GetFocus.vi"() -> ("error out"=w461:errorcluster, "dup hWnd"=w462:T1)  [unwired: 1 in, 9 out]
          n190 = call "GetWindowText.vi"("error in (no error)"=w461, "nMaxCount"=w458, "hWnd (NULL)"=w462) -> ("error out"=w459:errorcluster, "window text"=w460:string)  [unwired: 7 out]
        }
      }
      n191 = Unbundle By Name(w418) -> ("code"=w451:i32, "source"=w450:string)
      n192 = Unbundle By Name(w438) -> ("code"=w446:i32, "source"=w445:string)
      n193 = Unbundle By Name(w442) -> ("code"=w440:i32, "source"=w441:string)
      n194 = Format Into String(format string=w454, w451, w450, w449, w444, w446, w445, w439, w440, w441) -> (resulting string=w453:string)  [unwired: 2 in, 1 out]
    }
    frame 10 {
      w499 = 50 ("nMaxCount")
      # "Puts in front of\nbrowser"
      # "Setting the parent to NULL was really bizare.  THe client and panel were hidden on tray then when\nI showed the client both panels appeared."
      # "This refreshs"
      n195 = call "FindWindow.vi"("error in (no error)"=w493, "window name (\"\")"=w511) -> ("error out"=w504:errorcluster, "hWnd"=w503:T1)  [unwired: 6 out]
      n196 = call "GetForegroundWindow.vi"("error in (no error)"=w493) -> ("error out"=w492:errorcluster, "dup hWnd"=w479:T1)  [unwired: 9 out]
      n197 = call "GetWindowText.vi"("error in (no error)"=w504, "nMaxCount"=w499, "hWnd (NULL)"=w503) -> ("error out"=w489:errorcluster, "window text"=w505:string, "dup hWnd"=w491:T1)  [unwired: 6 out]
      n198 = call "U32 to hWnd.vi"("hWnd"=u32 0) -> ("hWnd"=w470:T1)  [unwired: 4 out]
      n199 = call "SetParent.vi"("error in (no error)"=w492, "hWndParent (NULL)"=w470, "hWndChild (NULL)"=w491) -> ("error out"=w490:errorcluster, "dup hWndChild"=w468:T1)  [unwired: 7 out]
      n200 = Merge Errors(w490, w489) -> (w488:errorcluster)
      n201 = call "SetWindowPos.vi"("Flags"=T3 {"SWP_NOSIZE (x1)"=TRUE, "SWP_NOMOVE (x2)"=TRUE, "SWP_NOZORDER (x4)"=FALSE, "SWP_NOREDRAW (x8)"=FALSE, "SWP_NOACTIVATE (x10)"=FALSE, "SWP_DRAWFRAME (x20)"=FALSE, "SWP_SHOWWINDOW (x40)"=FALSE, "SWP_HIDEWINDOW (x80)"=FALSE, "SWP_NOCOPYBITS (x100)"=FALSE, "SWP_NOOWNERZORDER (x200)"=FALSE, "SWP_NOSENDCHANGING (x400)"=FALSE, "SWP_DEFERERASE (x2000)"=FALSE, "SWP_ASYNCWINDOWPOS (x4000)"=FALSE}, "hWndInsertAfterALT\n(HWND_TOP)"=T4."HWND_TOPMOST" ("hWndInsertAfterALT\n(HWND_TOP)"), "error in (no error)"=w488, "hWndInsertAfter\n(NULL - use ALT)"=w479, "hWnd (NULL)"=w468) -> ("error out"=w482:errorcluster, "dup hWnd"=w483:T1)  [unwired: 1 in, 4 out]
      n202 = call "ShowWindow.vi"("error in (no error)"=w482, "nCmdShow\n(SW_SHOWNORMAL)"=T2."SW_FORCEMINIMIZE" ("nCmdShow\n(SW_SHOWNORMAL)"), "hWnd (NULL)"=w483) -> ("error out"=w487:errorcluster, "dup hWnd"=w486:T1)  [unwired: 7 out]
      n203 = call "ShowWindow.vi"("error in (no error)"=w487, "nCmdShow\n(SW_SHOWNORMAL)"=T2."SW_SHOWMAXIMIZED" ("nCmdShow\n(SW_SHOWNORMAL)"), "hWnd (NULL)"=w486) -> ("error out"=w476:errorcluster, "dup hWnd"=w478:T1)  [unwired: 7 out]
      n204 = call "ShowWindow.vi"("error in (no error)"=w476, "nCmdShow\n(SW_SHOWNORMAL)"=T2."SW_SHOWNORMAL" ("nCmdShow\n(SW_SHOWNORMAL)"), "hWnd (NULL)"=w478) -> ("error out"=w472:errorcluster, "dup hWnd"=w477:T1)  [unwired: 7 out]
      n205 = stacked-sequence {
        tunnel: "Yo" -> [_]
        tunnel: w472 -> [w512]
        tunnel: [w512] -> w471
        frame #0 {
        }
      }
      n206 = call "SetFocus.vi"("error in (no error)"=w471, "hWnd (NULL)"=w477) -> ("error out"=w474:errorcluster, "dup hWnd"=w481:T1)  [unwired: 8 out]
      n207 = stacked-sequence {
        tunnel: w499 -> [w521]
        tunnel: [w519] -> w500
        tunnel: [w518] -> w494
        tunnel: w474 -> [_]
        frame #0 {
          n208 = call "GetForegroundWindow.vi"() -> ("error out"=w520:errorcluster, "dup hWnd"=w522:T1)  [unwired: 1 in, 9 out]
          n209 = call "GetWindowText.vi"("error in (no error)"=w520, "nMaxCount"=w521, "hWnd (NULL)"=w522) -> ("error out"=w518:errorcluster, "window text"=w519:string)  [unwired: 7 out]
        }
      }
      n210 = stacked-sequence {
        tunnel: [w513] -> _
        tunnel: [w515] -> w495
        tunnel: [w514] -> w498
        tunnel: w499 -> [w513]
        tunnel: w474 -> [_]
        frame #0 {
          n211 = call "GetFocus.vi"() -> ("error out"=w516:errorcluster, "dup hWnd"=w517:T1)  [unwired: 1 in, 9 out]
          n212 = call "GetWindowText.vi"("error in (no error)"=w516, "nMaxCount"=w513, "hWnd (NULL)"=w517) -> ("error out"=w514:errorcluster, "window text"=w515:string)  [unwired: 7 out]
        }
      }
      n213 = Unbundle By Name(w474) -> ("code"=w507:i32, "source"=w506:string)
      n214 = Unbundle By Name(w494) -> ("code"=w502:i32, "source"=w501:string)
      n215 = Unbundle By Name(w498) -> ("code"=w496:i32, "source"=w497:string)
      n216 = Format Into String(format string=w510, w507, w506, w505, w500, w502, w501, w495, w496, w497) -> (resulting string=w509:string)  [unwired: 2 in, 1 out]
    }
    frame 11 {
      # "Puts in front of\nbrowser"
      # "Setting the parent to NULL was really bizare.  THe client and panel were hidden on tray then when\nI showed the client both panels appeared."
      # "This refreshs"
      n217 = Open VI Reference(vi path="Spartan Client.vi") -> (vi reference=w535:refnum<vi>, error out=w530:errorcluster)  [unwired: 1 in, 4 out]
      n218 = call "FindWindow.vi"("error in (no error)"=w533, "window name (\"\")"=w574) -> ("error out"=w567:errorcluster, "hWnd"=w566:T1)  [unwired: 6 out]
      n219 = property class="VI"(reference=w535, error in=w530) -> (reference out=w527:refnum<vi>, error out=w529:errorcluster, "Front Panel Window:Title"=w534:string)
      n220 = call "GetWindowText.vi"("error in (no error)"=w567, "nMaxCount"=50, "hWnd (NULL)"=w566) -> ("error out"=w532:errorcluster, "window text"=w568:string, "dup hWnd"=w556:T1)  [unwired: 6 out]
      n221 = call "FindWindow.vi"("error in (no error)"=w533, "window name (\"\")"=w534) -> ("error out"=w526:errorcluster, "hWnd"=w525:T1)  [unwired: 6 out]
      n222 = Close Reference(reference=w527, error in (no error)=w529) -> (error out=w528:errorcluster)
      n223 = call "GetForegroundWindow.vi"("error in (no error)"=w532) -> ("error out"=w531:errorcluster, "dup hWnd"=w524:T1)  [unwired: 9 out]
      n224 = call "SetParent.vi"("error in (no error)"=w526, "hWndParent (NULL)"=w524, "hWndChild (NULL)"=w525) -> ("error out"=w523:errorcluster)  [unwired: 8 out]
      n225 = call "SetParent.vi"("error in (no error)"=w523, "hWndParent (NULL)"=w524, "hWndChild (NULL)"=w556) -> ("error out"=w555:errorcluster, "dup hWndChild"=w537:T1)  [unwired: 7 out]
      n226 = Merge Errors(w555, w531, w528) -> (w554:errorcluster)
      n227 = call "SetWindowPos.vi"("Flags"=T3 {"SWP_NOSIZE (x1)"=TRUE, "SWP_NOMOVE (x2)"=TRUE, "SWP_NOZORDER (x4)"=FALSE, "SWP_NOREDRAW (x8)"=FALSE, "SWP_NOACTIVATE (x10)"=FALSE, "SWP_DRAWFRAME (x20)"=FALSE, "SWP_SHOWWINDOW (x40)"=FALSE, "SWP_HIDEWINDOW (x80)"=FALSE, "SWP_NOCOPYBITS (x100)"=FALSE, "SWP_NOOWNERZORDER (x200)"=FALSE, "SWP_NOSENDCHANGING (x400)"=FALSE, "SWP_DEFERERASE (x2000)"=FALSE, "SWP_ASYNCWINDOWPOS (x4000)"=FALSE}, "hWndInsertAfterALT\n(HWND_TOP)"=T4."HWND_TOPMOST" ("hWndInsertAfterALT\n(HWND_TOP)"), "error in (no error)"=w554, "hWndInsertAfter\n(NULL - use ALT)"=w524, "hWnd (NULL)"=w537) -> ("error out"=w548:errorcluster, "dup hWnd"=w549:T1)  [unwired: 1 in, 4 out]
      n228 = call "ShowWindow.vi"("error in (no error)"=w548, "nCmdShow\n(SW_SHOWNORMAL)"=T2."SW_FORCEMINIMIZE" ("nCmdShow\n(SW_SHOWNORMAL)"), "hWnd (NULL)"=w549) -> ("error out"=w553:errorcluster, "dup hWnd"=w552:T1)  [unwired: 7 out]
      n229 = call "ShowWindow.vi"("error in (no error)"=w553, "nCmdShow\n(SW_SHOWNORMAL)"=T2."SW_SHOWMAXIMIZED" ("nCmdShow\n(SW_SHOWNORMAL)"), "hWnd (NULL)"=w552) -> ("error out"=w543:errorcluster, "dup hWnd"=w545:T1)  [unwired: 7 out]
      n230 = call "ShowWindow.vi"("error in (no error)"=w543, "nCmdShow\n(SW_SHOWNORMAL)"=T2."SW_SHOWNORMAL" ("nCmdShow\n(SW_SHOWNORMAL)"), "hWnd (NULL)"=w545) -> ("error out"=w539:errorcluster, "dup hWnd"=w544:T1)  [unwired: 7 out]
      n231 = stacked-sequence {
        tunnel: "Yo" -> [_]
        tunnel: w539 -> [w575]
        tunnel: [w575] -> w538
        frame #0 {
        }
      }
      n232 = call "SetFocus.vi"("error in (no error)"=w538, "hWnd (NULL)"=w544) -> ("error out"=w541:errorcluster, "dup hWnd"=w547:T1)  [unwired: 8 out]
      n233 = stacked-sequence {
        tunnel: [w583] -> w563
        tunnel: [w582] -> w557
        tunnel: w541 -> [_]
        frame #0 {
          n234 = call "GetForegroundWindow.vi"() -> ("error out"=w584:errorcluster, "dup hWnd"=w585:T1)  [unwired: 1 in, 9 out]
          n235 = call "GetWindowText.vi"("error in (no error)"=w584, "nMaxCount"=50, "hWnd (NULL)"=w585) -> ("error out"=w582:errorcluster, "window text"=w583:string)  [unwired: 7 out]
        }
      }
      n236 = stacked-sequence {
        tunnel: [w578] -> w558
        tunnel: [w577] -> w561
        tunnel: [w576] -> _
        tunnel: w541 -> [_]
        frame #0 {
          w576 = 50 ("nMaxCount")
          n237 = call "GetFocus.vi"() -> ("error out"=w579:errorcluster, "dup hWnd"=w580:T1)  [unwired: 1 in, 9 out]
          n238 = call "GetWindowText.vi"("error in (no error)"=w579, "nMaxCount"=w576, "hWnd (NULL)"=w580) -> ("error out"=w577:errorcluster, "window text"=w578:string)  [unwired: 7 out]
        }
      }
      n239 = Unbundle By Name(w541) -> ("code"=w570:i32, "source"=w569:string)
      n240 = Unbundle By Name(w557) -> ("code"=w565:i32, "source"=w564:string)
      n241 = Unbundle By Name(w561) -> ("code"=w559:i32, "source"=w560:string)
      n242 = Format Into String(format string=w573, w570, w569, w568, w563, w565, w564, w558, w559, w560) -> (resulting string=w572:string)  [unwired: 2 in, 1 out]
    }
    frame 12 {
      w587 = T4."HWND_TOPMOST" ("hWndInsertAfterALT\n(HWND_TOP)")
      # "Puts in front of\nbrowser"
      # "The browser minimixed then I maxed it still the vi was not focused."
      # "This refreshs"
      n243 = Open VI Reference(vi path="Spartan Client.vi") -> (vi reference=w603:refnum<vi>, error out=w599:errorcluster)  [unwired: 1 in, 4 out]
      n244 = call "FindWindow.vi"("error in (no error)"=w601, "window name (\"\")"=w640) -> ("error out"=w634:errorcluster, "hWnd"=w633:T1)  [unwired: 6 out]
      n245 = property class="VI"(reference=w603, error in=w599) -> (reference out=w596:refnum<vi>, error out=w598:errorcluster, "Front Panel Window:Title"=w602:string)
      n246 = call "GetWindowText.vi"("error in (no error)"=w634, "nMaxCount"=50, "hWnd (NULL)"=w633) -> ("error out"=w600:errorcluster, "window text"=w635:string, "dup hWnd"=w623:T1)  [unwired: 6 out]
      n247 = call "FindWindow.vi"("error in (no error)"=w601, "window name (\"\")"=w602) -> ("error out"=w595:errorcluster, "hWnd"=w594:T1)  [unwired: 6 out]
      n248 = Close Reference(reference=w596, error in (no error)=w598) -> (error out=w597:errorcluster)
      n249 = call "GetForegroundWindow.vi"("error in (no error)"=w600) -> ("error out"=w589:errorcluster, "dup hWnd"=w590:T1)  [unwired: 9 out]
      n250 = call "SetWindowPos.vi"("hWndInsertAfterALT\n(HWND_TOP)"=w587, "error in (no error)"=w589, "hWnd (NULL)"=w590) -> ("error out"=w588:errorcluster, "dup hWnd"=w586:T1)  [unwired: 3 in, 4 out]
      n251 = call "SetWindowPos.vi"("hWndInsertAfterALT\n(HWND_TOP)"=T4."HWND_TOPMOST" ("hWndInsertAfterALT\n(HWND_TOP)"), "error in (no error)"=w595, "hWnd (NULL)"=w594) -> ("error out"=w591:errorcluster)  [unwired: 3 in, 5 out]
      n252 = call "SetParent.vi"("error in (no error)"=w588, "hWndParent (NULL)"=w586, "hWndChild (NULL)"=w623) -> ("error out"=w592:errorcluster, "dup hWndChild"=w605:T1)  [unwired: 7 out]
      n253 = Merge Errors(w592, w591, w597) -> (w622:errorcluster)
      n254 = call "SetWindowPos.vi"("Flags"=T3 {"SWP_NOSIZE (x1)"=TRUE, "SWP_NOMOVE (x2)"=TRUE, "SWP_NOZORDER (x4)"=FALSE, "SWP_NOREDRAW (x8)"=FALSE, "SWP_NOACTIVATE (x10)"=FALSE, "SWP_DRAWFRAME (x20)"=FALSE, "SWP_SHOWWINDOW (x40)"=FALSE, "SWP_HIDEWINDOW (x80)"=FALSE, "SWP_NOCOPYBITS (x100)"=FALSE, "SWP_NOOWNERZORDER (x200)"=FALSE, "SWP_NOSENDCHANGING (x400)"=FALSE, "SWP_DEFERERASE (x2000)"=FALSE, "SWP_ASYNCWINDOWPOS (x4000)"=FALSE}, "hWndInsertAfterALT\n(HWND_TOP)"=w587, "error in (no error)"=w622, "hWndInsertAfter\n(NULL - use ALT)"=w586, "hWnd (NULL)"=w605) -> ("error out"=w616:errorcluster, "dup hWnd"=w617:T1)  [unwired: 1 in, 4 out]
      n255 = call "ShowWindow.vi"("error in (no error)"=w616, "nCmdShow\n(SW_SHOWNORMAL)"=T2."SW_FORCEMINIMIZE" ("nCmdShow\n(SW_SHOWNORMAL)"), "hWnd (NULL)"=w617) -> ("error out"=w621:errorcluster, "dup hWnd"=w620:T1)  [unwired: 7 out]
      n256 = call "ShowWindow.vi"("error in (no error)"=w621, "nCmdShow\n(SW_SHOWNORMAL)"=T2."SW_SHOWMAXIMIZED" ("nCmdShow\n(SW_SHOWNORMAL)"), "hWnd (NULL)"=w620) -> ("error out"=w611:errorcluster, "dup hWnd"=w613:T1)  [unwired: 7 out]
      n257 = call "ShowWindow.vi"("error in (no error)"=w611, "nCmdShow\n(SW_SHOWNORMAL)"=T2."SW_SHOWNORMAL" ("nCmdShow\n(SW_SHOWNORMAL)"), "hWnd (NULL)"=w613) -> ("error out"=w607:errorcluster, "dup hWnd"=w612:T1)  [unwired: 7 out]
      n258 = stacked-sequence {
        tunnel: "Yo" -> [_]
        tunnel: w607 -> [w641]
        tunnel: [w641] -> w606
        frame #0 {
        }
      }
      n259 = call "SetFocus.vi"("error in (no error)"=w606, "hWnd (NULL)"=w612) -> ("error out"=w609:errorcluster, "dup hWnd"=w615:T1)  [unwired: 8 out]
      n260 = stacked-sequence {
        tunnel: [w649] -> w630
        tunnel: [w648] -> w624
        tunnel: w609 -> [_]
        frame #0 {
          n261 = call "GetForegroundWindow.vi"() -> ("error out"=w650:errorcluster, "dup hWnd"=w651:T1)  [unwired: 1 in, 9 out]
          n262 = call "GetWindowText.vi"("error in (no error)"=w650, "nMaxCount"=50, "hWnd (NULL)"=w651) -> ("error out"=w648:errorcluster, "window text"=w649:string)  [unwired: 7 out]
        }
      }
      n263 = stacked-sequence {
        tunnel: [w644] -> w625
        tunnel: [w643] -> w628
        tunnel: [w642] -> _
        tunnel: w609 -> [_]
        frame #0 {
          w642 = 50 ("nMaxCount")
          n264 = call "GetFocus.vi"() -> ("error out"=w645:errorcluster, "dup hWnd"=w646:T1)  [unwired: 1 in, 9 out]
          n265 = call "GetWindowText.vi"("error in (no error)"=w645, "nMaxCount"=w642, "hWnd (NULL)"=w646) -> ("error out"=w643:errorcluster, "window text"=w644:string)  [unwired: 7 out]
        }
      }
      n266 = Unbundle By Name(w609) -> ("code"=w637:i32, "source"=w636:string)
      n267 = Unbundle By Name(w624) -> ("code"=w632:i32, "source"=w631:string)
      n268 = Unbundle By Name(w628) -> ("code"=w626:i32, "source"=w627:string)
      n269 = Format Into String(format string=w639, w637, w636, w635, w630, w632, w631, w625, w626, w627) -> (resulting string=w638:string)  [unwired: 2 in, 1 out]
    }
    frame 13 {
      # "Puts in front of\nbrowser"
      # "The browser minimixed then I maxed it still the vi was not focused.\n\nThe client cannot be shown when marked topmost"
      # "This refreshs"
      n270 = Open VI Reference(vi path="Spartan Client.vi") -> (vi reference=w667:refnum<vi>, error out=w663:errorcluster)  [unwired: 1 in, 4 out]
      n271 = call "FindWindow.vi"("error in (no error)"=w665, "window name (\"\")"=w704) -> ("error out"=w698:errorcluster, "hWnd"=w697:T1)  [unwired: 6 out]
      n272 = property class="VI"(reference=w667, error in=w663) -> (reference out=w660:refnum<vi>, error out=w662:errorcluster, "Front Panel Window:Title"=w666:string)
      n273 = call "GetWindowText.vi"("error in (no error)"=w698, "nMaxCount"=50, "hWnd (NULL)"=w697) -> ("error out"=w664:errorcluster, "window text"=w699:string, "dup hWnd"=w687:T1)  [unwired: 6 out]
      n274 = call "FindWindow.vi"("error in (no error)"=w665, "window name (\"\")"=w666) -> ("error out"=w659:errorcluster, "hWnd"=w658:T1)  [unwired: 6 out]
      n275 = Close Reference(reference=w660, error in (no error)=w662) -> (error out=w661:errorcluster)
      n276 = call "GetForegroundWindow.vi"("error in (no error)"=w664) -> ("error out"=w653:errorcluster, "dup hWnd"=w652:T1)  [unwired: 9 out]
      n277 = call "SetWindowPos.vi"("hWndInsertAfterALT\n(HWND_TOP)"=T4."HWND_TOPMOST" ("hWndInsertAfterALT\n(HWND_TOP)"), "error in (no error)"=w659, "hWnd (NULL)"=w658) -> ("error out"=w655:errorcluster)  [unwired: 3 in, 5 out]
      n278 = call "SetParent.vi"("error in (no error)"=w653, "hWndParent (NULL)"=w652, "hWndChild (NULL)"=w687) -> ("error out"=w656:errorcluster, "dup hWndChild"=w669:T1)  [unwired: 7 out]
      n279 = Merge Errors(w656, w655, w661) -> (w686:errorcluster)
      n280 = call "SetWindowPos.vi"("Flags"=T3 {"SWP_NOSIZE (x1)"=TRUE, "SWP_NOMOVE (x2)"=TRUE, "SWP_NOZORDER (x4)"=FALSE, "SWP_NOREDRAW (x8)"=FALSE, "SWP_NOACTIVATE (x10)"=FALSE, "SWP_DRAWFRAME (x20)"=FALSE, "SWP_SHOWWINDOW (x40)"=FALSE, "SWP_HIDEWINDOW (x80)"=FALSE, "SWP_NOCOPYBITS (x100)"=FALSE, "SWP_NOOWNERZORDER (x200)"=FALSE, "SWP_NOSENDCHANGING (x400)"=FALSE, "SWP_DEFERERASE (x2000)"=FALSE, "SWP_ASYNCWINDOWPOS (x4000)"=FALSE}, "hWndInsertAfterALT\n(HWND_TOP)"=T4."HWND_TOPMOST" ("hWndInsertAfterALT\n(HWND_TOP)"), "error in (no error)"=w686, "hWndInsertAfter\n(NULL - use ALT)"=w652, "hWnd (NULL)"=w669) -> ("error out"=w680:errorcluster, "dup hWnd"=w681:T1)  [unwired: 1 in, 4 out]
      n281 = call "ShowWindow.vi"("error in (no error)"=w680, "nCmdShow\n(SW_SHOWNORMAL)"=T2."SW_FORCEMINIMIZE" ("nCmdShow\n(SW_SHOWNORMAL)"), "hWnd (NULL)"=w681) -> ("error out"=w685:errorcluster, "dup hWnd"=w684:T1)  [unwired: 7 out]
      n282 = call "ShowWindow.vi"("error in (no error)"=w685, "nCmdShow\n(SW_SHOWNORMAL)"=T2."SW_SHOWMAXIMIZED" ("nCmdShow\n(SW_SHOWNORMAL)"), "hWnd (NULL)"=w684) -> ("error out"=w675:errorcluster, "dup hWnd"=w677:T1)  [unwired: 7 out]
      n283 = call "ShowWindow.vi"("error in (no error)"=w675, "nCmdShow\n(SW_SHOWNORMAL)"=T2."SW_SHOWNORMAL" ("nCmdShow\n(SW_SHOWNORMAL)"), "hWnd (NULL)"=w677) -> ("error out"=w671:errorcluster, "dup hWnd"=w676:T1)  [unwired: 7 out]
      n284 = stacked-sequence {
        tunnel: "Yo" -> [_]
        tunnel: w671 -> [w705]
        tunnel: [w705] -> w670
        frame #0 {
        }
      }
      n285 = call "SetFocus.vi"("error in (no error)"=w670, "hWnd (NULL)"=w676) -> ("error out"=w673:errorcluster, "dup hWnd"=w679:T1)  [unwired: 8 out]
      n286 = stacked-sequence {
        tunnel: [w713] -> w694
        tunnel: [w712] -> w688
        tunnel: w673 -> [_]
        frame #0 {
          n287 = call "GetForegroundWindow.vi"() -> ("error out"=w714:errorcluster, "dup hWnd"=w715:T1)  [unwired: 1 in, 9 out]
          n288 = call "GetWindowText.vi"("error in (no error)"=w714, "nMaxCount"=50, "hWnd (NULL)"=w715) -> ("error out"=w712:errorcluster, "window text"=w713:string)  [unwired: 7 out]
        }
      }
      n289 = stacked-sequence {
        tunnel: [w708] -> w689
        tunnel: [w707] -> w692
        tunnel: [w706] -> _
        tunnel: w673 -> [_]
        frame #0 {
          w706 = 50 ("nMaxCount")
          n290 = call "GetFocus.vi"() -> ("error out"=w709:errorcluster, "dup hWnd"=w710:T1)  [unwired: 1 in, 9 out]
          n291 = call "GetWindowText.vi"("error in (no error)"=w709, "nMaxCount"=w706, "hWnd (NULL)"=w710) -> ("error out"=w707:errorcluster, "window text"=w708:string)  [unwired: 7 out]
        }
      }
      n292 = Unbundle By Name(w673) -> ("code"=w701:i32, "source"=w700:string)
      n293 = Unbundle By Name(w688) -> ("code"=w696:i32, "source"=w695:string)
      n294 = Unbundle By Name(w692) -> ("code"=w690:i32, "source"=w691:string)
      n295 = Format Into String(format string=w703, w701, w700, w699, w694, w696, w695, w689, w690, w691) -> (resulting string=w702:string)  [unwired: 2 in, 1 out]
    }
    frame 14 {
      # "Puts in front of\nbrowser"
      # "This refreshs"
      n296 = Open VI Reference(vi path="Spartan Client.vi") -> (vi reference=w728:refnum<vi>, error out=w724:errorcluster)  [unwired: 1 in, 4 out]
      n297 = call "FindWindow.vi"("error in (no error)"=w726, "window name (\"\")"=w765) -> ("error out"=w759:errorcluster, "hWnd"=w758:T1)  [unwired: 6 out]
      n298 = property class="VI"(reference=w728, error in=w724) -> (reference out=w721:refnum<vi>, error out=w723:errorcluster, "Front Panel Window:Title"=w727:string)
      n299 = call "GetWindowText.vi"("error in (no error)"=w759, "nMaxCount"=50, "hWnd (NULL)"=w758) -> ("error out"=w725:errorcluster, "window text"=w760:string, "dup hWnd"=w748:T1)  [unwired: 6 out]
      n300 = call "FindWindow.vi"("error in (no error)"=w726, "window name (\"\")"=w727) -> ("error out"=w716:errorcluster)  [unwired: 7 out]
      n301 = Close Reference(reference=w721, error in (no error)=w723) -> (error out=w722:errorcluster)
      n302 = call "GetForegroundWindow.vi"("error in (no error)"=w725) -> ("error out"=w718:errorcluster, "dup hWnd"=w717:T1)  [unwired: 9 out]
      n303 = call "SetParent.vi"("error in (no error)"=w718, "hWndParent (NULL)"=w717, "hWndChild (NULL)"=w748) -> ("error out"=w720:errorcluster, "dup hWndChild"=w730:T1)  [unwired: 7 out]
      n304 = Merge Errors(w720, w716, w722) -> (w747:errorcluster)
      n305 = call "SetWindowPos.vi"("Flags"=T3 {"SWP_NOSIZE (x1)"=TRUE, "SWP_NOMOVE (x2)"=TRUE, "SWP_NOZORDER (x4)"=FALSE, "SWP_NOREDRAW (x8)"=FALSE, "SWP_NOACTIVATE (x10)"=FALSE, "SWP_DRAWFRAME (x20)"=FALSE, "SWP_SHOWWINDOW (x40)"=FALSE, "SWP_HIDEWINDOW (x80)"=FALSE, "SWP_NOCOPYBITS (x100)"=FALSE, "SWP_NOOWNERZORDER (x200)"=FALSE, "SWP_NOSENDCHANGING (x400)"=FALSE, "SWP_DEFERERASE (x2000)"=FALSE, "SWP_ASYNCWINDOWPOS (x4000)"=FALSE}, "hWndInsertAfterALT\n(HWND_TOP)"=T4."HWND_TOPMOST" ("hWndInsertAfterALT\n(HWND_TOP)"), "error in (no error)"=w747, "hWndInsertAfter\n(NULL - use ALT)"=w717, "hWnd (NULL)"=w730) -> ("error out"=w741:errorcluster, "dup hWnd"=w742:T1)  [unwired: 1 in, 4 out]
      n306 = call "ShowWindow.vi"("error in (no error)"=w741, "nCmdShow\n(SW_SHOWNORMAL)"=T2."SW_FORCEMINIMIZE" ("nCmdShow\n(SW_SHOWNORMAL)"), "hWnd (NULL)"=w742) -> ("error out"=w746:errorcluster, "dup hWnd"=w745:T1)  [unwired: 7 out]
      n307 = call "ShowWindow.vi"("error in (no error)"=w746, "nCmdShow\n(SW_SHOWNORMAL)"=T2."SW_SHOWMAXIMIZED" ("nCmdShow\n(SW_SHOWNORMAL)"), "hWnd (NULL)"=w745) -> ("error out"=w736:errorcluster, "dup hWnd"=w738:T1)  [unwired: 7 out]
      n308 = call "ShowWindow.vi"("error in (no error)"=w736, "nCmdShow\n(SW_SHOWNORMAL)"=T2."SW_SHOWNORMAL" ("nCmdShow\n(SW_SHOWNORMAL)"), "hWnd (NULL)"=w738) -> ("error out"=w732:errorcluster, "dup hWnd"=w737:T1)  [unwired: 7 out]
      n309 = stacked-sequence {
        tunnel: "Yo" -> [_]
        tunnel: w732 -> [w766]
        tunnel: [w766] -> w731
        frame #0 {
        }
      }
      n310 = call "SetFocus.vi"("error in (no error)"=w731, "hWnd (NULL)"=w737) -> ("error out"=w734:errorcluster, "dup hWnd"=w740:T1)  [unwired: 8 out]
      n311 = stacked-sequence {
        tunnel: [w774] -> w755
        tunnel: [w773] -> w749
        tunnel: w734 -> [_]
        frame #0 {
          n312 = call "GetForegroundWindow.vi"() -> ("error out"=w775:errorcluster, "dup hWnd"=w776:T1)  [unwired: 1 in, 9 out]
          n313 = call "GetWindowText.vi"("error in (no error)"=w775, "nMaxCount"=50, "hWnd (NULL)"=w776) -> ("error out"=w773:errorcluster, "window text"=w774:string)  [unwired: 7 out]
        }
      }
      n314 = stacked-sequence {
        tunnel: [w769] -> w750
        tunnel: [w768] -> w753
        tunnel: w734 -> [_]
        frame #0 {
          n315 = call "GetFocus.vi"() -> ("error out"=w770:errorcluster, "dup hWnd"=w771:T1)  [unwired: 1 in, 9 out]
          n316 = call "GetWindowText.vi"("error in (no error)"=w770, "nMaxCount"=50, "hWnd (NULL)"=w771) -> ("error out"=w768:errorcluster, "window text"=w769:string)  [unwired: 7 out]
        }
      }
      n317 = Unbundle By Name(w734) -> ("code"=w762:i32, "source"=w761:string)
      n318 = Unbundle By Name(w749) -> ("code"=w757:i32, "source"=w756:string)
      n319 = Unbundle By Name(w753) -> ("code"=w751:i32, "source"=w752:string)
      n320 = Format Into String(format string=w764, w762, w761, w760, w755, w757, w756, w750, w751, w752) -> (resulting string=w763:string)  [unwired: 2 in, 1 out]
    }
    frame 15 {
      w798 = 50 ("nMaxCount")
      # "Added switch"
      # "The window appears but does not refresh and does not get focus\noddly the window flashes, set fore failed with NULL\nbrowser = fore, vi = focus"
      n321 = call "FindWindow.vi"("error in (no error)"=w792, "window name (\"\")"=w810) -> ("error out"=w803:errorcluster, "hWnd"=w802:T1)  [unwired: 6 out]
      n322 = call "GetForegroundWindow.vi"("error in (no error)"=w792) -> ("error out"=w791:errorcluster, "dup hWnd"=w790:T1)  [unwired: 9 out]
      n323 = call "GetWindowText.vi"("error in (no error)"=w803, "nMaxCount"=w798, "hWnd (NULL)"=w802) -> ("error out"=w787:errorcluster, "window text"=w804:string, "dup hWnd"=w789:T1)  [unwired: 6 out]
      n324 = call "SetParent.vi"("error in (no error)"=w791, "hWndParent (NULL)"=w790, "hWndChild (NULL)"=w789) -> ("error out"=w788:errorcluster)  [unwired: 8 out]
      n325 = Merge Errors(w788, w787) -> (w786:errorcluster)
      n326 = call "SetWindowPos.vi"("Flags"=w785, "hWndInsertAfterALT\n(HWND_TOP)"=T4."HWND_TOPMOST" ("hWndInsertAfterALT\n(HWND_TOP)"), "error in (no error)"=w786, "hWnd (NULL)"=w789) -> ("error out"=w780:errorcluster, "dup hWnd"=w778:T1)  [unwired: 2 in, 4 out]
      n327 = call "SwitchtoThisWindow.vi"("error in (no error)"=w780, "hWnd (NULL)"=w778) -> ("error out"=w779:errorcluster, "dup hWnd"=w777:T1)  [unwired: 8 out]
      n328 = call "SetFocus.vi"("error in (no error)"=w779, "hWnd (NULL)"=w777) -> ("error out"=w784:errorcluster, "dup hWnd"=w783:T1)  [unwired: 8 out]
      n329 = call "SetForegroundWindow.vi"("error in (no error)"=w784, "hWnd (NULL)"=w783) -> ("error out"=w781:errorcluster, "dup hWnd"=w782:T1)  [unwired: 8 out]
      n330 = stacked-sequence {
        tunnel: w798 -> [w819]
        tunnel: [w817] -> w799
        tunnel: [w816] -> w793
        tunnel: w781 -> [_]
        frame #0 {
          n331 = call "GetForegroundWindow.vi"() -> ("error out"=w818:errorcluster, "dup hWnd"=w820:T1)  [unwired: 1 in, 9 out]
          n332 = call "GetWindowText.vi"("error in (no error)"=w818, "nMaxCount"=w819, "hWnd (NULL)"=w820) -> ("error out"=w816:errorcluster, "window text"=w817:string)  [unwired: 7 out]
        }
      }
      n333 = stacked-sequence {
        tunnel: [w811] -> _
        tunnel: [w813] -> w794
        tunnel: [w812] -> w797
        tunnel: w798 -> [w811]
        tunnel: w781 -> [_]
        frame #0 {
          n334 = call "GetFocus.vi"() -> ("error out"=w814:errorcluster, "dup hWnd"=w815:T1)  [unwired: 1 in, 9 out]
          n335 = call "GetWindowText.vi"("error in (no error)"=w814, "nMaxCount"=w811, "hWnd (NULL)"=w815) -> ("error out"=w812:errorcluster, "window text"=w813:string)  [unwired: 7 out]
        }
      }
      n336 = Unbundle By Name(w781) -> ("code"=w806:i32, "source"=w805:string)
      n337 = Unbundle By Name(w793) -> ("code"=w801:i32, "source"=w800:string)
      n338 = Unbundle By Name(w797) -> ("code"=w795:i32, "source"=w796:string)
      n339 = Format Into String(format string=w809, w806, w805, w804, w799, w801, w800, w794, w795, w796) -> (resulting string=w808:string)  [unwired: 2 in, 1 out]
    }
    frame 16 {
      w845 = 50 ("nMaxCount")
      # "The window appears but does not refresh and does not get focus\noddly the window flashes, set fore failed with NULL\nbrowser = fore, vi = focus"
      n340 = call "FindWindow.vi"("error in (no error)"=w839, "window name (\"\")"=w856) -> ("error out"=w850:errorcluster, "hWnd"=w849:T1)  [unwired: 6 out]
      n341 = call "GetForegroundWindow.vi"("error in (no error)"=w839) -> ("error out"=w836:errorcluster, "dup hWnd"=w838:T1)  [unwired: 9 out]
      n342 = call "GetWindowText.vi"("error in (no error)"=w850, "nMaxCount"=w845, "hWnd (NULL)"=w849) -> ("window text"=w851:string, "dup hWnd"=w830:T1)  [unwired: 7 out]
      n343 = call "ShowWindow.vi"("error in (no error)"=w836, "nCmdShow\n(SW_SHOWNORMAL)"=T2."SW_SHOWMAXIMIZED" ("nCmdShow\n(SW_SHOWNORMAL)"), "hWnd (NULL)"=w838) -> ("error out"=w834:errorcluster, "dup hWnd"=w835:T1)  [unwired: 1 in, 6 out]
      n344 = call "GetWindowThreadProcessId.vi"("error in (no error)"=w834, "hWnd (NULL)"=w835) -> ("error out"=w833:errorcluster, "threadID"=w825:u32)  [unwired: 8 out]
      n345 = call "GetcurrentThreadId.vi"("error in (no error)"=w833) -> ("error out"=w832:errorcluster, "threadID"=w824:u32)  [unwired: 9 out]
      n346 = call "AttachThreadInput.vi"("error in (no error)"=w832, "Fattach"=TRUE, "threadID attach"=w824, "threadID Attachto"=w825) -> ("error out"=w831:errorcluster)  [unwired: 7 out]
      n347 = call "SetForegroundWindow.vi"("error in (no error)"=w831, "hWnd (NULL)"=w830) -> ("error out"=w828:errorcluster, "dup hWnd"=w829:T1)  [unwired: 8 out]
      n348 = call "SetFocus.vi"("error in (no error)"=w828, "hWnd (NULL)"=w829) -> ("error out"=w826:errorcluster, "dup hWnd"=w821:T1)  [unwired: 8 out]
      n349 = call "AttachThreadInput.vi"("error in (no error)"=w826, "Fattach"=FALSE, "threadID attach"=w824, "threadID Attachto"=w825) -> ("error out"=w822:errorcluster)  [unwired: 7 out]
      n350 = stacked-sequence {
        tunnel: w845 -> [w865]
        tunnel: [w863] -> w846
        tunnel: [w862] -> w840
        tunnel: w822 -> [_]
        frame #0 {
          n351 = call "GetForegroundWindow.vi"() -> ("error out"=w864:errorcluster, "dup hWnd"=w866:T1)  [unwired: 1 in, 9 out]
          n352 = call "GetWindowText.vi"("error in (no error)"=w864, "nMaxCount"=w865, "hWnd (NULL)"=w866) -> ("error out"=w862:errorcluster, "window text"=w863:string)  [unwired: 7 out]
        }
      }
      n353 = stacked-sequence {
        tunnel: [w857] -> _
        tunnel: [w859] -> w841
        tunnel: [w858] -> w844
        tunnel: w845 -> [w857]
        tunnel: w822 -> [_]
        frame #0 {
          n354 = call "GetFocus.vi"() -> ("error out"=w860:errorcluster, "dup hWnd"=w861:T1)  [unwired: 1 in, 9 out]
          n355 = call "GetWindowText.vi"("error in (no error)"=w860, "nMaxCount"=w857, "hWnd (NULL)"=w861) -> ("error out"=w858:errorcluster, "window text"=w859:string)  [unwired: 7 out]
        }
      }
      n356 = Unbundle By Name(w822) -> ("code"=w853:i32, "source"=w852:string)
      n357 = Unbundle By Name(w840) -> ("code"=w848:i32, "source"=w847:string)
      n358 = Unbundle By Name(w844) -> ("code"=w842:i32, "source"=w843:string)
      n359 = Format Into String(format string=w855, w853, w852, w851, w846, w848, w847, w841, w842, w843) -> (resulting string=w854:string)  [unwired: 2 in, 1 out]
    }
  }
  "Window name" <- w8
  "hWnd reference" <- w4
  "dup VI Refnum" <- "VI Refnum"
